vi "eveDataConverter.vi"() -> ()   [LabVIEW 2019]
uses:
  <vilib>/Analysis/NI_AALBase.lvlib
panel:
  out "key sort":u32[](array[numeric])
  out "Value sort":u32[](array[numeric])
  out "Array 2":u32[](array[numeric])
  out "Counts (map)":map{u32, u32}(c390)
  out "Histogram Graph":T1(graph)
  out "Channel":u32[](array[numeric])
  out "Energy":u32[](array[numeric])
  out "Chan+Energy":u32[](array[numeric])
  out "Clk Ticks":u32[](array[numeric])
  out "Sr No":i32[](array[numeric])
  out "Array":string[](array[string])
  out "rsvd+partity":u32
  out "pha":u32
  out "channel":u32
  in  "Input Binary String":string
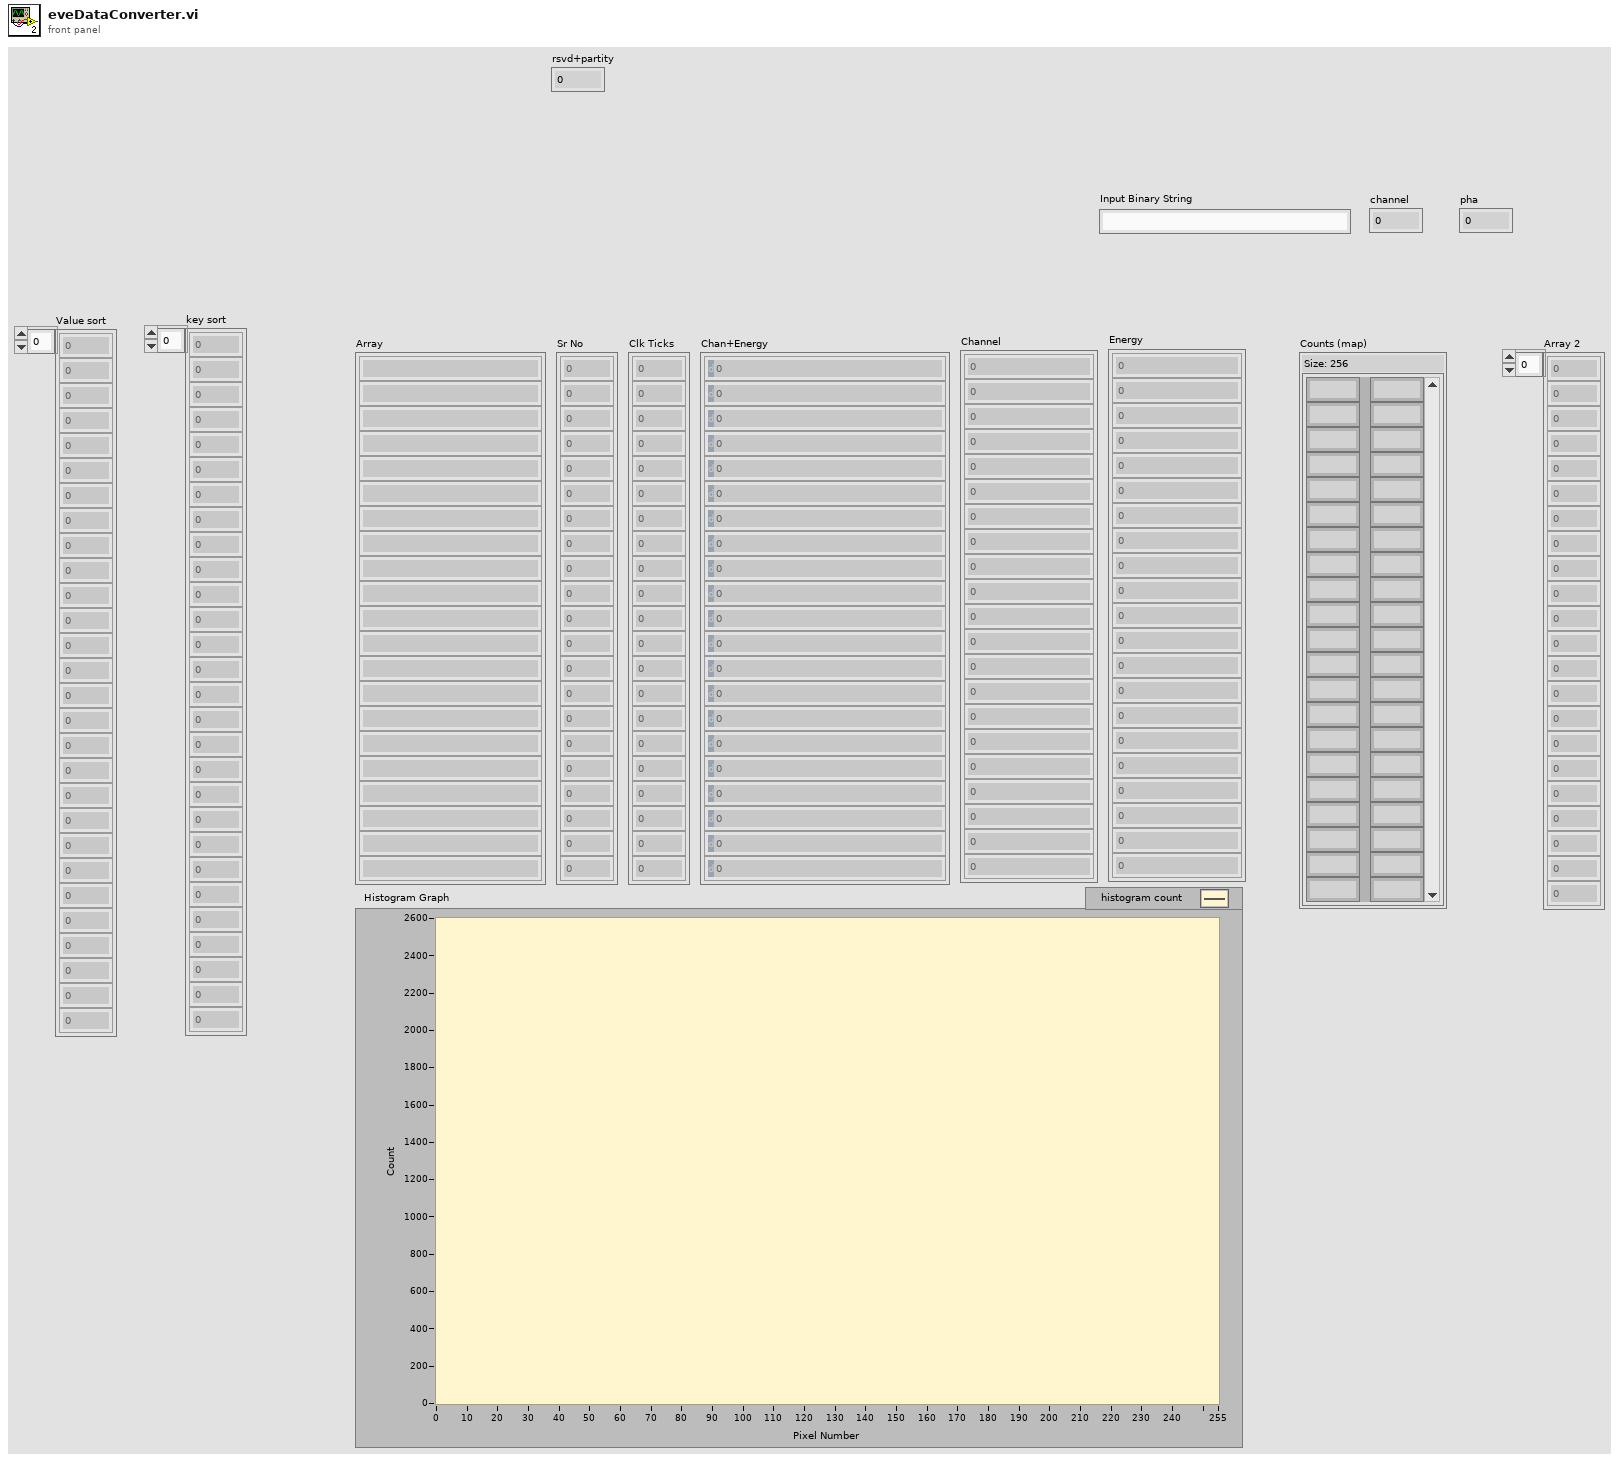
[diagram p1: front panel]
types:
  T1 = cluster{"X Values":dbl[], "Histogram: h(x)":i32[]}
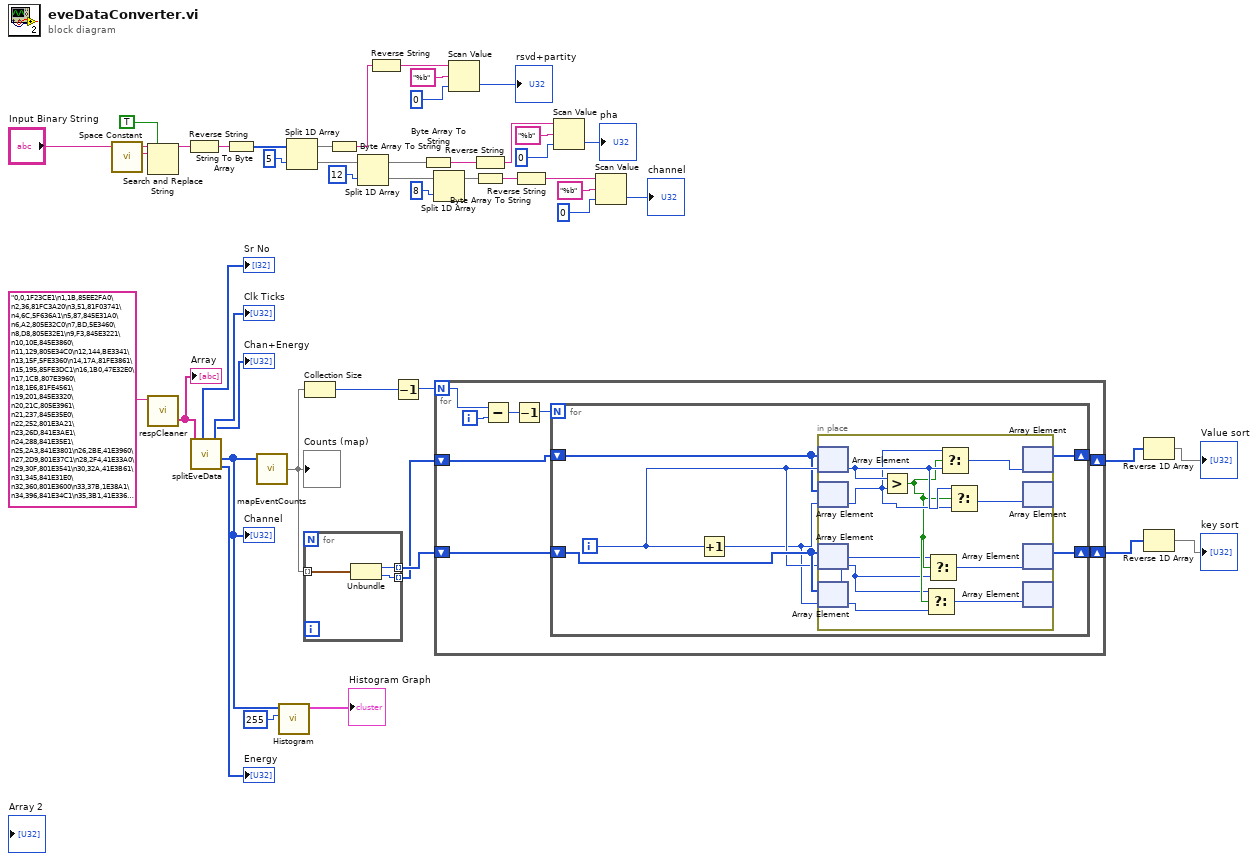
[diagram p0: block diagram]
diagram:
  n1 = call <vilib>:"Space Constant.vi"() -> ("String"=w46:string)
  n2 = Search and Replace String(replace all?=TRUE ("replace all? (F)"), input string="Input Binary String", search string=w46) -> (result string=w41:string)  [unwired: 5 in, 3 out]
  n3 = call "respCleaner.vi"("Raw Response"="0,0,1F23CE1\n1,1B,85EE2FA0\n2,36,81FC3A20\n3,51,81F03741\n4,6C,5F636A1\n5,87,845E31A0\n6,A2,805E32C0\n7,BD,5E3460\n8,D8,805E32E1\n9,F3,845E3221\n10,10E,845E3860\n11,129,805E34C0\n12,144,BE3341\n13,15F,5FE3360\n14,17A,81FE3861\n15,195,85FE3DC1\n16,1B0,47E32E0\n17,1CB,807E3960\n18,1E6,81FE4561\n19,201,845E3320\n20,21C,805E3961\n21,237,845E35E0\n22,252,801E3A21\n23,26D,841E3AE1\n24,288,841E35E1\n25,2A3,841E3801\n26,2BE,41E3960\n27,2D9,801E37C1\n28,2F4,41E33A0\n29,30F,801E3541\n30,32A,41E3B61\n31,345,841E31E0\n32,360,801E3600\n33,37B,1E38A1\n34,396,841E34C1\n35,3B1,41E3360\n36,3CC,801E37C1\n37,3E7,41E3500\n38,402,1E43C1\n39,41D,41E3C41\n40,438,41E36A0\n41,453,801E34C1\n42,46E,41E3541\n43,489,41E3941\n44,4A4,41E37A1\n45,4BF,841E3300\n46,4DA,1E36A0\n47,4F5,801E3880\n48,510,1E3440\n49,52B,1E3FC0\n50,546,1E3641\n51,561,41E3720\n52,57C,801E3720\n53,597,80BE32E0\n54,5B2,80BE35E1\n55,5CD,84BE3161\n56,5E8,84BE34C1\n57,603,4BE3220\n58,61E,80BE30C0\n59,639,1FE3240\n60,654,1FE33C0\n61,66F,7E3681\n62,68A,47E3921\n63,6A5,845E33C1\n64,6C0,45E31C0\n65,6DB,5E3D00\n66,6F6,BE3101\n67,711,4BE36E1\n68,72C,84BE3541\n69,747,5FE3140\n70,762,1FE2F61\n71,77D,85FE33A0\n72,798,81FE3401\n73,7B3,5FE3461\n74,7CE,847E35C0\n75,7E9,7E39A0\n76,804,805E34A0\n77,81F,805E2F81\n78,83A,45E31C0\n79,855,1E40E0\n80,870,801E3641\n81,88B,41E35E1\n82,8A6,841E3B61\n83,8C1,841E3600\n84,8DC,1E3360\n85,8F7,801E3880\n86,912,1E33C0\n87,92D,1E35E1\n88,948,841E35C0\n89,963,1E3960\n90,97E,801E3880\n91,999,1E3660\n92,9B4,801E3560\n93,9CF,801E2FE0\n94,9EA,801E38C1\n95,A05,41E3AC0\n96,A20,1E3560\n97,A3B,801E3AA0\n98,A56,801E3180\n99,A71,1E4380\n100,A8C,1E37A1\n101,AA7,841E40A1\n102,AC2,841E3D61\n103,ADD,84DE38E0\n104,AF8,801E37C1\n105,B13,41E33A0\n106,B2E,801E35E1\n107,B49,841E36C0\n108,B64,1E37C1\n109,B7F,41E3EE0\n110,B9A,801E3A00\n111,BB5,1E34A1\n112,BD0,841E37E0\n113,BEB,801E3C81\n114,C06,41E3CE1\n115,C21,841E3740\n116,C3C,1E3801\n117,C57,41E37E0\n118,C72,801E3521\n119,C8D,841E34C1\n120,CA8,45E2B01\n121,CC3,45E3501\n122,CDE,4BE3360\n123,CF9,80BE32C1\n124,D14,4BE3180\n125,D2F,BE3321\n126,D4A,85FE3740\n127,D65,1FE3201\n128,D80,5FE3261\n129,D9B,85FE30C0\n130,DB6,7E3820\n131,DD1,805E39E0\n132,DEC,80BE3201\n133,E07,4BE3321\n134,E22,84BE35A0\n135,E3D,80BE3261\n136,E58,84BE38A1\n137,E73,85FE3880\n138,E8E,1FE37A1\n139,EA9,85FE33C0\n140,EC4,7E3600\n141,EDF,7E3621\n142,EFA,845E3080\n143,F15,5E3221\n144,F30,841E39A0\n145,F4B,801E3701\n146,F66,41E32E0\n147,F81,801E3120\n148,F9C,801E3740\n149,FB7,1E3761\n150,FD2,841E34E0\n151,FED,801E36E1\n152,1008,841E3BE0\n153,1023,801E38E0\n154,103E,801E37E0\n155,1059,801E3801\n156,1074,41E3641\n157,108F,41E3720\n158,10AA,801E37E0\n159,10C5,801E3621\n160,10E0,841E3500\n161,10FB,1E3CA0\n162,1116,801E3761\n163,1131,841E3761\n164,114C,841E36C0\n165,1167,1E3621\n166,1182,841E3D40\n167,119D,1E3880\n168,11B8,1E35E1\n169,11D3,841E3BC1\n170,11EE,41E3420\n171,1209,801E36E1\n172,1224,841E3280\n173,123F,1E35C0\n174,125A,1E3AA0\n175,1275,80BE3420\n176,1290,80BE3000\n177,12AB,BE3300\n178,12C6,BE3300\n179,12E1,BE3560\n180,12FC,81FE3621\n181,1317,847E3461\n182,1332,845E3421\n183,134D,841E3381\n184,1368,41E37A1\n185,1383,845E3141\n186,139E,41E38E0\n187,13B9,801E35A0\n188,13D4,801E3C60\n189,13EF,801E37C1\n190,140A,41E3560\n191,1425,801E3EE0\n192,1440,801E36E1\n193,145B,841E35E1\n194,1476,841E35C0\n195,1491,1E3480\n196,14AC,1E3521\n197,14C7,841E33A0\n198,14E2,80BE31E0\n199,14FD,80BE32E0\n200,1518,80BE30A0\n201,1533,80BE3280\n202,154E,BE35A0\n203,1569,80BE3440\n204,1584,1FE3261\n205,159F,85FE31E0\n206,15BA,81FE3941\n207,15D5,47E35E1\n208,15F0,845E3481\n209,160B,45E3520\n210,1626,80BE3461\n211,1641,85FE3921\n212,165C,84BE3321\n213,1677,84BE3120\n214,1692,81FE33C0\n215,16AD,1FE3AA0\n216,16C8,81FE3921\n217,16E3,85FE39A0\n218,16FE,807E33E1\n219,1719,841E37E0\n220,1734,805E32A0\n221,174F,805E3160\n222,176A,805E32E1\n223,1785,841E3AE1\n224,17A0,845E3421\n225,17BB,84BE3461\n226,17D6,847E29A1\n227,17F1,84BE3461\n228,180C,84BE3461\n229,1827,85FE33C0\n230,1842,1FE4241\n231,185D,5FE3500\n232,1878,7E3560\n233,1893,805E35E0\n234,18AE,805E34A0\n235,18C9,80BE32A1\n236,18E4,84BE3201\n237,18FF,4BE3360\n238,191A,81FE33E1\n239,1935,85FE35E1\n240,1950,847E3480\n241,196B,5E36C1\n242,1986,45E3320\n243,19A1,805E3601\n244,19BC,4BE3201\n245,19D7,4BE3341\n246,19F2,4BE3480\n247,1A0D,1FE3761\n248,1A28,847E35A0\n249,1A43,81FE4400\n250,1A5E,5E3320\n251,1A79,805E3421\n252,1A94,84BE3541\n253,1AAF,4BE35A0\n254,1ACA,80BE3641\n255,1AE5,5FE3480\n256,1B00,1FE3541\n257,1B1B,5EC3581\n258,1B36,5F047C1\n259,1B51,5EE3800\n260,1B6C,1FA40A0\n261,1B87,81F445C1\n262,1BA2,5F83E20\n263,1BBD,81F64140\n264,1BD8,1FC4180\n265,1BF3,1F24BC0\n266,1C0E,DE39A0\n267,1C29,81FE6EA1\n268,1C44,85FE38A1\n269,1C5F,85FE36C0\n270,1C7A,1FE3600\n271,1C95,1FE30E1\n272,1CB0,85FE3AE1\n273,1CCB,85FE3C21\n274,1CE6,85FE34C1\n275,1D01,5FE37E0\n276,1D1C,81FE4020\n277,1D37,80DE32C1\n278,1D52,5FE4301\n279,1D6D,5FE3D01\n280,1D88,5FE4881\n281,1DA3,47E38E0\n282,2870,1803060\n283,2949,1802EA0\n284,2DE8,1803021\n285,2E93,1803300\n286,39C8,5E32E1\n287,3DEB,1E36E1\n288,3FB2,1E3861\n289,3FE3,1E3A00\n290,402C,DE32C1\n291,405D,1E3B01\n292,40DC,1E41A0\n293,4125,1E3420\n294,4168,1E40E0\n295,41A7,1E3641\n296,41DA,1E38E0\n297,420B,1E3A60\n298,4248,1E3AA0\n299,427D,1E3E01\n300,42B0,DE33E1\n301,42E1,D03460\n302,4314,1E4221\n303,4345,DE3780\n304,4378,1E3560\n305,43CD,1E3801\n306,4400,1E3D61\n307,443F,1E47E1\n308,4472,DE3900\n309,44A9,1E4C01\n310,44E6,1E3CC0\n311,4551,1E3DE0\n312,7E94,BE3101\n313,7FBB,BE3381\n314,835C,1E4B81\n315,8475,1E3740\n316,84F8,1E3921\n317,853F,1E36E1\n318,95CA,5E3301\n319,10427,1FE3581\n320,10472,DE3000\n321,104A3,1FE3A60\n322,104F4,1FE37A1\n323,10543,1FE34C1\n324,10592,1FE3660\n325,1B345,BE3261\n326,1B38E,BE33A0\n327,3218F,1FE3480\n328,321C2,1FE34C1\n329,32211,1FE40A1\n330,32244,1FE3381\n331,3228F,1FE4340\n332,322DE,1FE4620\n333,32329,7E35A0\n334,3235C,1FE4EC0\n335,32395,1FE3861\n336,323C8,DE32A1\n337,323F9,1FE35C0\n338,3242C,7E3720\n339,3245D,1FE34A1\n340,32490,7E3780\n341,324C1,1FE3641\n342,32530,1FE4BA0\n343,34D23,5E3121\n344,34EA4,5E30A1\n345,34F51,5E30E0\n346,34FB0,5E26A0\n347,350A1,5E34A0\n348,35F3A,1E3C00\n349,35FE1,1E35E1\n350,3602A,1E36E1\n351,36073,1E3801\n352,360BC,1E3DC1\n353,36163,1E37A1\n354,361AA,1E3CA0\n355,361F1,1E3440\n356,3623A,1E3E61\n357,36281,1E4100\n358,362BC,1E4080\n359,36305,1E36A0\n360,36338,1E3681\n361,36387,1E35A0\n362,363E4,1E3BE0\n363,36421,1E3681\n364,36470,1E4760\n365,364A5,1E37A1\n366,364EE,1E43C1\n367,36535,1E3C21\n368,36574,1E3981\n369,365DB,1E3780\n370,3662C,1E3C81\n371,36661,1E3461\n372,366B2,1E3F00\n373,366F9,1E3861\n374,3672C,1E3A60\n375,36775,1E3321\n376,367A8,1E3C81\n377,367E1,1E3FA0\n378,368E2,1E34E0\n379,36965,1E37E0\n380,36998,1E4540\n381,36A1D,1E3720\n382,36B62,1E3960\n383,36BFD,1E3BC1\n384,36C68,1E3740\n385,36DD5,1E39A0\n386,36E3A,1E3000\n387,36EAB,1E36A0\n388,36EDE,1E3921\n389,36F0F,DE3880\n390,36F42,1E3F00\n391,36F7B,1E38A1\n392,36FB8,1E3641\n393,36FE9,1E3021\n394,37038,DE3C41\n395,370A7,1E42A0\n396,37104,1E3220\n397,3730D,1E3740\n398,3737C,1E35C0\n399,373FD,1E3C00\n400,37466,1E37A1\n401,37637,1E3B61\n402,3767E,1E35C0\n403,376C7,1E3F21\n404,3778C,1E36A0\n405,377D3,1E35A0\n406,37844,1E3BE0\n407,3794D,1E3440\n408,379BE,1E37A1\n409,37A07,1E43C1\n410,37A3A,1E33C0\n411,37A79,1E3820\n412,37AC2,1E38A1\n413,37B09,1E3F41\n414,37B3C,1E3AA0\n415,37B8B,1E38C1\n416,37BC0,1E3960\n417,37BF1,1E3A21\n418,37C40,DE3521\n419,37C87,1E3A21\n420,37CBA,1E35A0\n421,37D03,1E3A00\n422,37D36,1E34E0\n423,37DDB,1E33E1\n424,38C72,BE33C0\n425,38D5F,BE33C0\n426,48DBE,BE30A0\n427,48E69,BE3600\n428,48EE6,BE3180\n429,4902B,BE34E0\n430,49072,BE33C0\n431,4927B,BE3360\n432,62FC4,1FE3521\n433,63011,7E3A41\n434,63044,1FE36A0\n435,63075,7E3560\n436,630A8,1FE3461\n437,630DF,1FE3DC1\n438,63114,1FE38E0\n439,63149,1FE3CA0\n440,6317C,DE3F41\n441,631AD,1FE3C00\n442,631E4,1FE3D20\n443,63217,1FE5060\n444,6324C,1FE3F21\n445,63299,DE36A0\n446,65BB6,5E33C1\n447,65C47,5E3320\n448,65DBA,5E3680\n449,66105,1E3981\n450,6630C,1E4020\n451,6633D,1E3420\n452,6644A,1E3701\n453,6647B,1E33C0\n454,664F8,1E3581\n455,66529,1E3360\n456,6657A,1E3820\n457,665C3,1E3AE1\n458,66632,1E37A1\n459,66679,1E38C1\n460,666C2,1E3F00\n461,666FD,1E3B61\n462,66730,1E4200\n463,66783,1E3DE0\n464,667B6,1E3780\n465,66805,1E40C1\n466,6685A,1E37C1\n467,668A1,1E3D80\n468,668FA,1E3CC0\n469,66931,1E3A81\n470,6697A,1E3A81\n471,669B1,1E3900\n472,669FC,1E42E1\n473,66A79,1E4421\n474,66AF4,1E3BC1\n475,66B31,1E4121\n476,69040,1E3581\n477,69181,1E3BE0\n478,691FA,1E3D20\n479,6925B,1E3A81\n480,6928E,1E3500\n481,69331,1E3461\n482,69CAA,BE33C0\n483,6A3E7,5E3221\n484,6A5A0,5E3260\n485,71B01,1FE3541\n486,71B4A,1FE3E80\n487,71B91,1FE34C1\n488,71BD8,1FE3701\n489,79D19,BE3180\n490,79DF0,BE3120\n491,93B05,1FE3420\n492,93B46,1FE3440\n493,93B8D,1FE4040\n494,93BD8,1FE3D01\n495,93C23,1FE3440\n496,93C56,1FE38A1\n497,93C95,1FE32E0\n498,93CC8,1FE3981\n499,93CF9,DE3B61\n500,93D2C,1FE3761\n501,93D63,1FE3CE1\n502,93D96,7E3280\n503,93DC7,1FE3BA1\n504,93E1A,DE34E0\n505,93E4B,1FE46C1\n506,96888,5E3281\n507,96B85,5E3481\n508,96BD8,5E3741\n509,971F3,1E3B20\n510,97226,1E3720\n511,97303,1E3B61\n512,9734C,1E33E1\n513,97393,1E3B80\n514,9741E,1E3321\n515,9745D,1E3581\n516,974A6,1E3900\n517,974E5,1E3480\n518,9755A,1E3480\n519,9758B,1E3C81\n520,975BE,DE30A0\n521,97607,1E3600\n522,97650,1E3581\n523,97681,1E3941\n524,976CC,1E40A1\n525,976FD,1E3381\n526,9774E,1E3880\n527,9777F,1E39A0\n528,977C8,1E4B41\n529,977F9,1E36A0\n530,97904,1E3541\n531,97935,1E3840\n532,97972,1E3740\n533,979B3,DE37A1\n534,979F2,1E4640\n535,97B1D,1E4241\n536,97D30,1E4181\n537,99A9F,1E3CA0\n538,99AD8,1E3440\n539,99B21,1E37E0\n540,99B5A,1E32E0\n541,99B8B,1E3581\n542,99BDA,1E3720\n543,99C23,1E3CC0\n544,99CAA,1E36A0\n545,99CF9,1E3541\n546,99D56,1E3B40\n547,9ABE7,BE3161\n548,9AC2A,BE3521\n549,9AC6D,BE3560\n550,9ACA2,BE3360\n551,A2907,1FE3F60\n552,A294A,1FE3681\n553,A297B,1FE3641\n554,A29C4,DE34A1\n555,A29F5,1FE3660\n556,AAD2E,BE33E1\n557,AAD9D,BE3600\n558,AAE54,BE3440\n559,C4991,1FE35A0\n560,C49DC,1FE4141\n561,C4A23,1FE43C1\n562,C4A62,1FE33A0\n563,C4AA9,1FE4481\n564,C4AF0,1FE40C1\n565,C4B21,1FE3060\n566,C4B54,1FE3641\n567,C4B8D,1FE3701\n568,C4BC0,7E3621\n569,C4BF1,1FE35E1\n570,C4C24,DE4260\n571,C4C55,1FE4481\n572,C4C90,1FE46C1\n573,C79E7,5E34E1\n574,C7B26,5E3380\n575,C7C0B,5E3421\n576,C7F12,1E3581\n577,C7F5B,1E3BC1\n578,C7FA4,1E3560\n579,C8163,1E3321\n580,C8196,1E35A0\n581,C81DD,1E3921\n582,C8210,1E39C0\n583,C8259,1E3E20\n584,C82A0,1E3C60\n585,C82E7,1E37E0\n586,C8330,1E4141\n587,C8371,1E35C0\n588,C83BA,1E3820\n589,C83F1,1E3A00\n590,C8492,1E3780\n591,C850D,1E39A0\n592,C8540,1E3B40\n593,C8581,1E39E1\n594,C85B8,1E3BA1\n595,C85FF,DE3DA1\n596,C8640,1E3921\n597,C8671,1E4200\n598,C8758,1E41E1\n599,C87AB,1E4281\n600,C8800,1E4260\n601,C8871,1E4181\n602,C8BCE,1E4901\n603,CA84D,1E3780\n604,CA8B8,1E35C0\n605,CA92F,1E3C00\n606,CA9A0,1E3B20\n607,CA9E7,DE3461\n608,CAA8C,1E47E1\n609,CAACB,1E3A41\n610,CAC60,1E37C1\n611,CB9A1,BE3360\n612,DB98C,BE3220\n613,DB9D7,BE3220\n614,DBAD0,BE3280\n615,F5513,1FE37A1\n616,F5562,1FE3A60\n617,F55B1,1FE3880\n618,F5600,1FE3480\n619,F564B,1FE3820\n620,F5696,1FE4141\n621,F56DD,1FE4EE1\n622,F5728,1FE3EA1\n623,F5773,1FE3EE0\n624,F57BC,1FE3861\n625,F57F5,1FE3461\n626,F5834,1FE35A0\n627,F5865,1FE3220\n628,F5898,DE3801\n629,F58C9,1FE35A0\n630,F58FC,7E33C0\n631,F592D,1FE3701\n632,F596C,1FE4281\n633,F599D,7E3641\n634,F59D0,1FE4260\n635,F5A01,DE3CA0\n636,F5A34,1FE4640\n637,F5A9D,1FE4561\n638,F842C,5E3020\n639,F85E1,5E3B81\n640,F8DAC,1E3861\n641,F931F,1E3701\n642,F9352,1E3BE0\n643,F947B,1E41C0\n644,F94AE,1E3641\n645,F9565,1E3B80\n646,F9598,1E3CA0\n647,F95D1,1E34C1\n648,F9612,1E3621\n649,F9661,1E4020\n650,F9694,1E3CE1\n651,F96EF,1E3560\n652,F974C,1E39E1\n653,F977D,1E3681\n654,F97C6,1E3A41\n655,F98B5,1E3681\n656,F991E,1E3CE1\n657,F999B,1E40A1\n658,F9A08,1E3F81\n659,F9A49,1E3C00\n660,F9A7C,1E41A0\n661,F9AAD,DE3820\n662,F9B22,1E3761\n663,F9B8B,1E3B01\n664,F9BD4,DE3541\n665,FA3B1,1E40C1\n666,FA578,1E3F41\n667,FA8A5,1E3660\n668,FA944,1E4540\n669,FA9AB,1E2C01\n670,FAB9E,1E3960\n671,FABCF,1E33A0\n672,FACB4,1E3621\n673,FAE2B,1E4221\n674,FAEA2,1E3A60\n675,FAF91,1E3420\n676,FB084,1E3820\n677,FB1AD,1E3FA0\n678,FB1E0,1E3660\n679,FB22F,1E3720\n680,FB39C,1E32E0\n681,FB52D,1E35A0\n682,FC632,BE37C1\n683,FC6A9,BE35A0\n684,10CCA2,BE3240\n685,10CDDB,BE3401\n686,10CF1C,BE3261\n687,10D5C7,BE3600\n688,1264F0,1FE3480\n689,126533,1FE3AC0\n690,12657E,1FE4721\n691,1265BF,1FE40E0\n692,1265F2,1FE3641\n693,126623,1FE3DA1\n694,126656,7E37A1\n695,126687,1FE39C0\n696,1266BA,DE3960\n697,1266EB,7E2CA1\n698,12671E,1FE4A20\n699,12676B,DE31C1\n700,129218,5E35A1\n701,129261,5E30E0\n702,1292C0,5E30C1\n703,129307,5E32A0\n704,129344,5E2F60\n705,129375,5E3520\n706,1293C4,5E3EC0\n707,129ACD,1E3740\n708,129C98,1E35C0\n709,129D47,1E3660\n710,129DA4,1E3CE1\n711,129F45,1E37C1\n712,12A020,1E3801\n713,12A05F,1E3681\n714,12A0A2,1E3C41\n715,12A0E9,1E44A0\n716,12A11C,1E3D80\n717,12A157,1E3761\n718,12A1A0,DE34E0\n719,12A1D1,1E38A1\n720,12A246,1E3820\n721,12A277,1E3F41\n722,12A2AA,1E3600\n723,12A2DB,1E3681\n724,12A30E,DE40E0\n725,12A33F,1E3DC1\n726,12A386,1E43A1\n727,12A465,1E3E61\n728,12A4AE,1E40C1\n729,12A4F7,1E40A1\n730,12A52A,1E3440\n731,12A56B,1E39A0\n732,12A5AE,DE3621\n733,12A611,1E41E1\n734,12A7D4,1E4460\n735,12B817,1E4680\n736,12B88C,1E35C0\n737,12BA43,1E41E1\n738,12BD38,1E3A60\n739,12BD7F,DE31E0\n740,12BDDC,1E36E1\n741,12BE0D,1E38A1\n742,12BE54,1E4141\n743,12BE85,1E3480\n744,12BECE,DE3BA1\n745,12BF29,1E3CA0\n746,12C094,1E33A0\n747,12C0DF,1E41E1\n748,12C134,1E3660\n749,12C165,1E3621\n750,12C1D2,1E3840\n751,12C219,1E3A81\n752,12C262,1E3660\n753,12C395,1E3820\n754,12C3C8,1E2A40\n755,12D3D1,BE32E0\n756,12D516,BE36C0\n757,12D585,BE3660\n758,13D95C,BE33E1\n759,13D9A3,BE36C0\n760,13DA4C,BE3A81\n761,13DAB9,BE31A1\n762,13DAFC,BE3941\n763,13DBB9,BE34E0\n764,13DCE8,BE31A1\n765,1571EF,1FE34C1\n766,157236,1FE3BA1\n767,157271,1FE3581\n768,1572BA,1FE4721\n769,1572EB,1FE3C81\n770,157326,1FE32E0\n771,157361,1FE3DA1\n772,1573AC,1FE4721\n773,1573DD,1FE3641\n774,157410,7E36A0\n775,157441,1FE4020\n776,157474,DE3701\n777,1574A5,1FE3761\n778,1574D8,7E3541\n779,157509,1FE41E1\n780,157554,DE36E1\n781,15A0C9,5E32C0\n782,15A11A,5E3340\n783,15A189,5E3281\n784,15A670,1E3C00\n785,15A76B,1E3740\n786,15A81A,1E35A0\n787,15AB7B,1E3A41\n788,15ACFA,1E3A41\n789,15AD3F,1E3E40\n790,15AD8E,1E3B20\n791,15ADEB,1E4320\n792,15AE36,1E48C0\n793,15AE7D,1E4821\n794,15AF08,1E35E1\n795,15AF57,1E3720\n796,15AF9A,1E3581\n797,15AFCB,1E3521\n798,15AFFE,1E3861\n799,15B02F,1E37C1\n800,15B066,1E39E1\n801,15B14B,1E3600\n802,15B1BC,1E39C0\n803,15B331,1E39E1\n804,15B364,1E3F00\n805,15B395,DE3341\n806,15B3C8,1E3761\n807,15B55F,1E5321\n808,15B606,1E4121\n809,15C907,1E3480\n810,15C94A,1E3A41\n811,15CAEB,1E4040\n812,15CC74,1E3F81\n813,15CD19,1E3541\n814,15CDB0,1E3B20\n815,15CDEF,1E41A0\n816,15CE22,1E35E1\n817,15CECB,1E35A0\n818,15CF1A,1E3CE1\n819,15CFB9,1E3A60\n820,15D054,1E3720\n821,15D091,1E3541\n822,15D16E,1E3740\n823,15D1B7,1E3621\n824,15D1FA,1E3480\n825,15E1BF,BE3420\n826,165EEC,1FE3521\n827,165F35,1FE3581\n828,165F86,1FE3960\n829,165FCF,1FE3381\n830,16E2F4,BE3401\n831,16E361,BE3BE0\n832,16E3A2,BE34A1\n833,16E455,BE3360\n834,187F58,1FE3381\n835,187FDD,1FE32E0\n836,188010,1FE32E0\n837,188041,1FE3681\n838,188074,7E3960\n839,1880A5,1FE3900\n840,1880D8,DE33E1\n841,188109,7E3801\n842,18813C,1FE3C41\n843,188177,1FE3C21\n844,1881AA,1FE36C0\n845,1881E3,1FE4AC1\n846,188216,DE4121\n847,18AEF3,5E31E1\n848,18AFE6,5E3441\n849,18B349,1E3440\n850,18B806,1E3AE1\n851,18B855,1E3541\n852,18BA0E,1E39A0\n853,18BAC1,1E3DE0\n854,18BB0A,1E4C01\n855,18BB5B,1E3720\n856,18BBB4,1E3401\n857,18BC01,1E3F81\n858,18BC44,1E37A1\n859,18BC8B,1E3B40\n860,18BCC6,1E3E40\n861,18BD15,1E3761\n862,18BD72,1E3D80\n863,18BDB9,1E37A1\n864,18BE0A,1E3900\n865,18BE3B,1E37A1\n866,18BE72,1E34C1\n867,18BEB3,1E3E40\n868,18BEE6,DE3500\n869,18BF17,1E3880\n870,18BF60,1E3960\n871,18BFA7,1E3F41\n872,18BFF0,1E3D61\n873,18C021,1E3720\n874,18C07A,1E3D01\n875,18C0FB,1E45A1\n876,18C168,1E3960\n877,18C1A7,1E3C41\n878,18C1DA,1E3AC0\n879,18CB95,1E4181\n880,18CDEA,1E45E0\n881,18CE1B,1E3BE0\n882,18D4E6,1E3780\n883,18D65B,1E3CA0\n884,18D6D6,1E4080\n885,18D71F,1E40A1\n886,18D762,1E3AC0\n887,18D793,1E37E0\n888,18D7CE,1E3BA1\n889,18D7FF,DE3740\n890,18D84E,1E3641\n891,18D895,1E4001\n892,18D8E8,1E3A21\n893,18D9D7,1E3600\n894,18DAA2,1E3521\n895,18DAE9,1E3381\n896,18DB3A,1E37A1\n897,18DBF3,1E3401\n898,18DCF6,1E3D40\n899,18DD3F,1E3621\n900,18DF58,1E38E0\n901,18EE57,BE3621\n902,18EEFC,BE3240\n903,18F3B5,5E3361\n904,1957C8,7E3480\n905,196C2B,1FE3440\n906,196CA2,1FE32E0\n907,196CF1,1FE3BE0\n908,196D40,1FE3B40\n909,19F45B,BE26A1\n910,19F4F6,BE3321\n911,19F563,BE3461\n912,19F5A6,BE31E0\n913,19F60F,BE3720\n914,19F78E,BE36E1\n915,19F8C5,BE36A0\n916,1B8D46,1FE37C1\n917,1B8DCB,1FE3401\n918,1B8E16,1FE4441\n919,1B8E47,1FE3C21\n920,1B8E90,1FE43A1\n921,1B8EC1,7E3401\n922,1B8EF4,1FE3C60\n923,1B8F2F,1FE3CC0\n924,1B8F62,1FE3B61\n925,1B8F93,DE3420\n926,1B8FC6,7E35E1\n927,1B8FF7,7E35C0\n928,1B902A,1FE4181\n929,1BBCC5,5E36E0\n930,1BC752,1E3600\n931,1BC845,1E43C1\n932,1BC88E,DE3440\n933,1BC8BF,1E4AA1\n934,1BC8FC,1E33C0\n935,1BC945,1E34E0\n936,1BCA0C,1E38C1\n937,1BCA3D,1E35A0\n938,1BCA9A,1E3681\n939,1BCACB,1E3780\n940,1BCB52,1E3740\n941,1BCBA9,1E36E1\n942,1BCBEC,1E3740\n943,1BCC35,1E38A1\n944,1BCC68,1E4260\n945,1BCCA3,1E3D20\n946,1BCCE6,1E3F00\n947,1BCD2D,1E3941\n948,1BCD76,1E3E20\n949,1BCDB1,1E37A1\n950,1BCDE4,1E35E1\n951,1BCE15,1E3861\n952,1BCE8E,1E38C1\n953,1BCECD,1E3C21\n954,1BCF0E,DE3E80\n955,1BCF3F,1E4800\n956,1BCF78,1E3820\n957,1BCFC7,1E3FA0\n958,1BD008,1E3FA0\n959,1BD075,1E3A60\n960,1BD15A,1E4061\n961,1BD1D1,1E3480\n962,1BD4DA,1E3D40\n963,1BE20F,1E34C1\n964,1BE2B6,1E46C1\n965,1BE2FD,1E3BE0\n966,1BE34C,1E3F00\n967,1BE4C5,1E29E0\n968,1BE578,1E34E0\n969,1BE5D5,1E2301\n970,1BE646,1E3780\n971,1BE8EF,1E3401\n972,1BE9AE,1E3B61\n973,1BEA2D,1E3C41\n974,1BFC1C,BE3921\n975,1BFC67,BE31E0\n976,1BFCD4,BE3420\n977,1BFD09,BE31E0\n978,1BFD52,DE34C1\n979,1BFF8F,5E31E1\n980,1C794C,1FE3C21\n981,1C7991,1FE3541\n982,1C79D8,1FE4281\n983,1CFE85,BE3A00\n984,1CFF72,BE23E0\n985,1CFFEB,BE3440\n986,1D002E,BE3EE0\n987,1E9817,1FE34C1\n988,1E999C,1FE35A0\n989,1E99E3,1FE3420\n990,1E9A32,1FE3B61\n991,1E9A7B,1FE48C0\n992,1E9AC4,1FE3BE0\n993,1E9AF5,1FE3521\n994,1E9B3C,1FE4281\n995,1E9B71,1FE34E0\n996,1E9BBA,1FE4901\n997,1E9BEB,1FE39E1\n998,1E9C26,7E3360\n999,1E9C57,1FE3E40\n1000,1E9C8A,DE39C0\n1001,1E9CBB,1FE3801\n1002,1E9CF6,1FE4CA1\n1003,1E9D27,1FE4241\n1004,1E9D76,DE35E1\n1005,1EC8EB,5E32C0\n1006,1ECA26,5E31A0\n1007,1ED2DB,1E3780\n1008,1ED318,1E3820\n1009,1ED521,1E36A0\n1010,1ED56E,1E3461\n1011,1ED5BD,1E3701\n1012,1ED658,1E3801\n1013,1ED6A9,1E37C1\n1014,1ED6EC,1E3500\n1015,1ED733,1E3941\n1016,1ED77A,1E3820\n1017,1ED7C1,1E3D40\n1018,1ED808,1E3600\n1019,1ED839,1E3C00\n1020,1ED884,1E4221\n1021,1ED8B5,1E3FC0\n1022,1ED8FC,DE3BE0\n1023,1ED92D,1E3D61\n1024,1ED97E,1E44E1\n1025,1ED9AF,1E34E0\n1026,1ED9EC,1E40A1\n1027,1EDA57,1E44A0\n1028,1EDB88,1E3A81\n1029,1EDBCF,1E4940\n1030,1EDCE4,1E3D20\n1031,1EDD4B,1E4501\n1032,1EDDA4,1E3C00\n1033,1EDE23,1E3F81\n1034,1EF576,1E3A81\n1035,1EF60B,1E3621\n1036,1EF662,1E3621\n1037,1EF6A9,1E3401\n1038,1EF6F0,1E3E20\n1039,1EF739,1E40E0\n1040,1EF78C,1E38E0\n1041,1EF7D5,1E3880\n1042,1EF818,1E36A0\n1043,1EF8CD,1E3DC1\n1044,1EF942,1E3560\n1045,1EFA6B,1E3FC0\n1046,1F09D0,BE31E0\n1047,1F0A49,BE3280\n1048,1F0C10,5E3320\n1049,200F13,BE3801\n1050,2011A6,BE3280\n1051,201215,BE3060\n1052,201322,BE3060\n1053,21A811,1FE3CE1\n1054,21A85C,1FE3720\n1055,21A8A5,1FE40A1\n1056,21A8DA,1FE3101\n1057,21A919,1FE37A1\n1058,21A94C,1FE3960\n1059,21A989,1FE3880\n1060,21A9BC,7E34C1\n1061,21A9ED,1FE3880\n1062,21AA20,DE38A1\n1063,21AA51,7E3C00\n1064,21AA84,1FE4DA0\n1065,21AAB9,1FE4700\n1066,21D696,5E3781\n1067,21D6CB,5E3380\n1068,21D714,DE3981\n1069,21DE53,1E3500\n1070,21DE9C,1E3560\n1071,21DED7,1E3600\n1072,21E018,1E37E0\n1073,21E067,1E3941\n1074,21E0AC,1E3C21\n1075,21E1D3,1E3820\n1076,21E21E,1E3AA0\n1077,21E261,1E4020\n1078,21E35A,1E4DC0\n1079,21E3A1,1E3440\n1080,21E3E8,1E4181\n1081,21E425,1E4421\n1082,21E48E,1E36A0\n1083,21E4D5,1E3740\n1084,21E514,1E39A0\n1085,21E563,1E5220\n1086,21E650,1E44C0\n1087,21E835,1E48E1\n1088,21FF30,1E3A21\n1089,2202AB,1E34C1\n1090,220316,1E3960\n1091,2203EB,1E3D80\n1092,2204DA,1E3461\n1093,220547,1E3641\n1094,220644,1E37C1\n1095,2206E5,1E3660\n1096,22072E,1E3681\n1097,220783,1E36C0\n1098,2207CC,1E35C0\n1099,2217DB,BE33E1\n1100,22184C,BE3521\n1101,229391,1FE38E0\n1102,231A50,BE3220\n1103,231A97,BE32C1\n1104,231AD6,BE3420\n1105,231B81,BE35C0\n1106,231CDE,BE3060\n1107,231E1F,BE3261\n1108,24B666,1FE31C1\n1109,24B697,7E3360\n1110,24B6DE,1FE4F40\n1111,24B70F,7E34A1\n1112,24B742,1FE34A1\n1113,24B777,1FE3A21\n1114,24B7B6,1FE3A41\n1115,24B7E7,DE4760\n1116,24B81A,1FE3BE0\n1117,24B853,1FE4221\n1118,24B8BC,1FE39A0\n1119,24E661,5E3821\n1120,24E6F0,5E3520\n1121,24EA0F,1E3541\n1122,24EBCC,1E3C81\n1123,24ED9D,1E3E80\n1124,24EDE0,1E3F81\n1125,24EE21,DE32C1\n1126,24EE54,1E3341\n1127,24EE85,1E3480\n1128,24EEC8,1E3660\n1129,24EF31,1E3C60\n1130,24EF7A,1E3840\n1131,24EFC3,1E3D61\n1132,24F00C,1E3541\n1133,24F03D,1E4181\n1134,24F0E0,1E3780\n1135,24F117,1E35A0\n1136,24F15E,1E3720\n1137,24F18F,1E3B61\n1138,24F1CC,1E3BA1\n1139,24F1FD,DE3E61\n1140,24F230,1E3E40\n1141,24F297,1E4001\n1142,24F306,1E3DC1\n1143,24F3D7,1E3C41\n1144,24F4C2,1E43C1\n1145,2512C7,1E3600\n1146,25133A,1E4380\n1147,25157D,1E3A41\n1148,2516C4,1E3941\n1149,251743,1E3AE1\n1150,2517E0,1E3840\n1151,252461,BE3401\n1152,25250C,5E32C0\n1153,25254F,BE3861\n1154,2525BA,5E3320\n1155,25A035,1FE3EE0\n1156,25A0C4,1FE36C0\n1157,25A10D,1FE4800\n1158,25A154,1FE3AE1\n1159,25A19B,1FE37C1\n1160,25A1E4,1FE36A0\n1161,262B0B,BE3401\n1162,262B54,BE3C81\n1163,262C03,BE32C1\n1164,262C72,BE3201\n1165,262D5F,BE3201\n1166,262EB8,BE3321\n1167,27C2AF,1FE3321\n1168,27C2F8,1FE4E81\n1169,27C335,1FE3461\n1170,27C37E,1FE43A1\n1171,27C3AF,1FE3DA1\n1172,27C3EC,1FE3981\n1173,27C421,1FE3420\n1174,27C454,DE3F21\n1175,27C485,1FE40C1\n1176,27C4B8,7E3621\n1177,27C4E9,1FE3880\n1178,27C51C,DE34C1\n1179,27C553,1FE39E1\n1180,27C586,1FE4961\n1181,27C5B7,DE3F60\n1182,27EE48,5E3281\n1183,27F01D,5E33A1\n1184,27F894,1E35C0\n1185,27FA0F,1E32E0\n1186,27FA50,1E36A0\n1187,27FC0D,1E3D01\n1188,27FC40,1E3681\n1189,27FCBB,1E37E0\n1190,27FCEE,1E3681\n1191,27FD1F,1E36C0\n1192,27FD52,DE42A0\n1193,27FD83,1E47E1\n1194,27FDBC,1E33E1\n1195,27FE03,1E37A1\n1196,27FE4A,1E3581\n1197,27FE87,1E3C60\n1198,27FED0,1E4061\n1199,27FF01,1E39C0\n1200,27FF98,1E3960\n1201,27FFE1,1E39C0\n1202,28004A,1E3DC1\n1203,28007B,1E4281\n1204,2800BC,1E36E1\n1205,280163,1E3C60\n1206,2801AC,1E4380\n1207,28029D,1E3C00\n1208,28048E,1E3341\n1209,281DAB,1E3461\n1210,281FE8,1E37A1\n1211,282031,1E3381\n1212,282064,1E3720\n1213,282095,1E38A1\n1214,2820C8,1E40E0\n1215,2820F9,DE4001\n1216,28212C,1E44C0\n1217,28323B,BE3060\n1218,283284,BE31C1\n1219,2832FB,BE3060\n1220,292FE4,BE3840\n1221,293095,BE39A0\n1222,2931F0,BE34A1\n1223,29332F,BE3560\n1224,29348E,BE3140\n1225,2935E1,BE3180\n1226,29373C,BE3180\n1227,2ACF3F,1FE3780\n1228,2ACF72,1FE2A01\n1229,2ACFA3,1FE3C21\n1230,2ACFEC,1FE4C20\n1231,2AD01D,1FE3641\n1232,2AD068,1FE3A81\n1233,2AD099,1FE3960\n1234,2AD0CC,DE3761\n1235,2AD0FD,1FE36E1\n1236,2AD148,1FE48C0\n1237,2AD179,1FE3600\n1238,2AD1BA,1FE4141\n1239,2AD1EB,1FE3720\n1240,2AD21E,7E34A1\n1241,2AD24F,1FE3D80\n1242,2AD282,DE43E0\n1243,2AD2B3,7E3461\n1244,2AFE44,5E34C0\n1245,2B0747,1E3681\n1246,2B07F4,1E3660\n1247,2B083B,DE30C0\n1248,2B086E,1E3AE1\n1249,2B08CB,1E38A1\n1250,2B0978,1E3341\n1251,2B09FB,1E3D01\n1252,2B0AC8,1E3720\n1253,2B0B0F,1E3921\n1254,2B0B4C,1E3900\n1255,2B0B7D,1E37C1\n1256,2B0BB0,1E4640\n1257,2B0C0B,1E39E1\n1258,2B0C46,1E3861\n1259,2B0C8B,1E35A0\n1260,2B0CBE,1E3621\n1261,2B0D15,1E3480\n1262,2B0D48,1E3761\n1263,2B0D83,1E41A0\n1264,2B0DB6,DE34A1\n1265,2B0E39,1E3541\n1266,2B0E74,1E39A0\n1267,2B0EBD,DE33E1\n1268,2B0F18,1E3921\n1269,2B105B,1E4040\n1270,2B10B8,1E3D01\n1271,2B284B,1E4561\n1272,2B2A38,1E3981\n1273,2B2B65,1E3641\n1274,2B2BC2,1E3D40\n1275,2B2D53,1E3500\n1276,2B2E68,1E34A1\n1277,2B2EAF,1E3941\n1278,2B2EE4,1E3C00\n1279,2B2F31,1E3A21\n1280,2B2F90,1E3B40\n1281,2B2FD9,1E34E0\n1282,2B300E,1E2A20\n1283,2B305D,1E3C81\n1284,2B30CA,1E36E1\n1285,2B3E5F,BE3440\n1286,2BBC44,1FE3341\n1287,2BBC8B,1FE3621\n1288,2BBCDA,1FE4061\n1289,2C49F5,BE3600\n1290,2C4B46,BE3261\n1291,2DDDB1,1FE32C1\n1292,2DDDFA,1FE4640\n1293,2DDE37,1FE3720\n1294,2DDE7E,1FE4561\n1295,2DDEAF,1FE3541\n1296,2DDEEC,1FE38C1\n1297,2DDF1F,1FE3280\n1298,2DDF52,7E3761\n1299,2DDF83,1FE3621\n1300,2DDFB6,DE33C0\n1301,2DDFE7,1FE3D20\n1302,2DE01A,7E3B61\n1303,2DE04B,1FE4580\n1304,2DE086,1FE4080\n1305,2DE0D1,DE3381\n1306,2E0C0C,5E3340\n1307,2E0C57,5E31E1\n1308,2E0CC6,5E33C1\n1309,2E11EB,1E31C1\n1310,2E1302,1E3641\n1311,2E1333,1E3780\n1312,2E1366,DE3440\n1313,2E13B5,1E3A00\n1314,2E1468,1E37C1\n1315,2E1499,1E3261\n1316,2E14CC,1E3861\n1317,2E150F,1E3420\n1318,2E1556,1E3880\n1319,2E159D,1E45C1\n1320,2E15D0,1E4400\n1321,2E1625,1E4281\n1322,2E1658,1E39A0\n1323,2E16B5,1E3461\n1324,2E16F6,1E3DA1\n1325,2E173D,1E48E1\n1326,2E1786,1E3B61\n1327,2E17CF,1E35A0\n1328,2E1810,1E3EA1\n1329,2E1857,DE33A0\n1330,2E18F8,1E37A1\n1331,2E1929,1E39A0\n1332,2E1962,1E37E0\n1333,2E1993,1E3E61\n1334,2E19C6,DE3FA0\n1335,2E19F7,1E3F81\n1336,2E1A34,1E38C1\n1337,2E1A77,1E3921\n1338,2E1AAA,1E4380\n1339,2E1AF3,DE3621\n1340,2E1BF2,1E39C0\n1341,2E1D2D,1E3981\n1342,2E1D9E,1E4441\n1343,2E1EB1,1E42E1\n1344,2E32A2,1E49E0\n1345,2E3A61,1E2F01\n1346,2E3C32,1E3681\n1347,2E3CA3,1E37E0\n1348,2E3CD6,1E34A1\n1349,2E3D1D,1E3581\n1350,2E3D66,1E3960\n1351,2E3E5B,1E3780\n1352,2E3ECE,1E3A00\n1353,2E3F21,1E3000\n1354,2E4D5A,BE3541\n1355,2F438F,BE33C0\n1356,2F4442,BE3401\n1357,2F4481,BE3F21\n1358,2F468A,BE3801\n1359,2F4805,BE3461\n1360,2F484C,1FE3401\n1361,2F487D,BE3420\n1362,30EA78,1FE31C1\n1363,30EAC1,1FE3DC1\n1364,30EAFC,1FE3A21\n1365,30EB3F,1FE37E0\n1366,30EB72,1FE3500\n1367,30EBB3,7E3300\n1368,30EBE6,1FE47A0\n1369,30EC17,DE4001\n1370,30EC4A,1FE3461\n1371,30EC7B,7E3D20\n1372,30ECAE,1FE3C60\n1373,30ECDF,7E3CA0\n1374,30ED18,1FE3B20\n1375,30ED5D,DE36A0\n1376,30EDC8,1FE3FE1\n1377,311B25,5E32E1\n1378,311D94,1E3880\n1379,31200F,1E36C0\n1380,312098,1E3541\n1381,3122DD,1E3220\n1382,312326,1E37E0\n1383,312371,1E3440\n1384,3123BA,1E32E0\n1385,31241B,1E39E1\n1386,312454,1E3AA0\n1387,312559,1E3740\n1388,312594,1E3801\n1389,3125E3,1E3701\n1390,31261C,1E3AE1\n1391,31264D,1E3BE0\n1392,312680,DE3AC0\n1393,3126B1,1E3C21\n1394,3126E4,1E3A60\n1395,31271D,1E3861\n1396,312760,1E4460\n1397,312791,1E3C41\n1398,3127C4,DE36A0\n1399,312805,1E36E1\n1400,31284E,1E3921\n1401,312895,1E4501\n1402,3128C8,1E3880\n1403,3128FF,1E3801\n1404,312946,1E3DC1\n1405,3129A3,1E3960\n1406,312A12,1E36E1\n1407,312B63,1E37C1\n1408,312C84,1E3DC1\n1409,312EDD,1E4481\n1410,314022,1E4361\n1411,3143A1,1E4061\n1412,3143D4,1E3C21\n1413,314423,1E36A0\n1414,31446C,1E42E1\n1415,3144B3,1E3AE1\n1416,31451E,1E2A40\n1417,31454F,1E3820\n1418,3145F4,1E3521\n1419,314671,1E33C0\n1420,3146F8,1E3981\n1421,31473F,1E45C1\n1422,31477A,1E3461\n1423,3147AF,1E3801\n1424,3147F8,1E3CE1\n1425,314847,1E4160\n1426,3148C2,1E37A1\n1427,314973,1E3401\n1428,315B36,BE3261\n1429,315BA7,BE32A1\n1430,326224,BE2DC0\n1431,32630D,BE3000\n1432,326350,BE3261\n1433,326427,BE33C0\n1434,33F772,1FE31A1\n1435,33F85D,1FE34A1\n1436,33F8A6,1FE3941\n1437,33F8ED,1FE3F21\n1438,33F936,7E3560\n1439,33F967,1FE5021\n1440,33F9A0,1FE3280\n1441,33F9D9,1FE3F60\n1442,33FA0C,DE34E0\n1443,33FA3D,1FE3801\n1444,33FA70,7E3B20\n1445,33FAA1,1FE3641\n1446,33FAD4,7E3681\n1447,33FB05,1FE3CA0\n1448,33FB40,1FE5341\n1449,33FB71,DE3581\n1450,34274A,5E30A1\n1451,34278B,5E3421\n1452,3427D6,5E32A0\n1453,342A6B,1E3581\n1454,342AB4,1802D21\n1455,342FFF,1E3861\n1456,343048,1E3621\n1457,34308B,1E3B01\n1458,34313C,1E3740\n1459,343179,1E3B20\n1460,3431AC,DE3AE1\n1461,3431DD,1E3621\n1462,343210,1E3360\n1463,343251,1E36C0\n1464,343292,1E39C0\n1465,3432CD,1E3500\n1466,343300,DE37E0\n1467,343331,1E3921\n1468,34337A,1E3921\n1469,3433AB,1E3500\n1470,3433F4,1E3A00\n1471,343493,1E45C1\n1472,3434C6,1E3761\n1473,3434FB,1E3960\n1474,343550,1E3BE0\n1475,3435AD,1E3840\n1476,343618,1E3921\n1477,34364D,1E3420\n1478,343684,1E3660\n1479,3436BF,1E3921\n1480,3436F2,DE43A1\n1481,343723,1E3CC0\n1482,34379C,1E3C60\n1483,343843,1E42C0\n1484,3438B4,1E4601\n1485,343D6F,1E50A0\n1486,3454FC,1E3641\n1487,345569,1E4061\n1488,345742,1E3D01\n1489,34577F,1E3E40\n1490,3457C8,1E3621\n1491,345843,1E3600\n1492,345894,1E3C41\n1493,3458DB,1E46C1\n1494,34590E,1E3720\n1495,345955,1E35E1\n1496,3459A4,1E3C41\n1497,3459DF,1E4020\n1498,3467DE,BE3560\n1499,346817,BE3740\n1500,34E3AE,1FE2680\n1501,34E3F7,1FE3E61\n1502,34E43E,1FE4400\n1503,34E485,1FE3960\n1504,356F5C,BE37C1\n1505,3570C9,BE3000\n1506,35720E,BE33A0\n1507,370469,1FE3720\n1508,37061C,1FE35E1\n1509,370667,1FE3D80\n1510,3706B0,1FE49C1\n1511,3706E1,1FE3621\n1512,370722,1FE36E1\n1513,370757,7E33C0\n1514,37078A,1FE3A00\n1515,3707BB,DE3880\n1516,3707EE,1FE3861\n1517,37082B,1FE3521\n1518,370896,1FE4D00\n1519,3734D1,5E32E1\n1520,373594,5E3481\n1521,37362D,5E3340\n1522,373D08,1E34A1\n1523,373DC9,1E3941\n1524,373E12,DE3341\n1525,373E43,1E35E1\n1526,373E76,1E37A1\n1527,373EBD,1E3801\n1528,373F08,1E3C00\n1529,373F65,1E3621\n1530,373F98,1E3461\n1531,373FD9,1E3740\n1532,374088,1E3300\n1533,3740C5,1E3A21\n1534,374104,1E3780\n1535,374135,1E3820\n1536,374168,1E3880\n1537,374199,1E3900\n1538,3741CC,DE31C1\n1539,3741FD,1E45E0\n1540,37424C,1E3621\n1541,374293,1E34A1\n1542,37435C,1E3F41\n1543,3743A3,1E4540\n1544,3743D6,1E3D80\n1545,374429,1E3641\n1546,374472,1E40A1\n1547,3744A3,1E3C00\n1548,3744D6,1E3101\n1549,374515,1E4501\n1550,374548,1E3F00\n1551,374583,1E43A1\n1552,3745CC,DE3AA0\n1553,374695,1E4661\n1554,3761B4,1E3CA0\n1555,37629D,1E3DE0\n1556,376336,1E3681\n1557,3763A7,1E3701\n1558,376464,1E34A1\n1559,3764CB,1E3600\n1560,37654C,1E3A00\n1561,3765BD,1E3280\n1562,3766BE,1E3780\n1563,3767FB,1E3440\n1564,37758E,BE34A1\n1565,377871,5E3800\n1566,37F1C0,1FE3E61\n1567,37F20F,1FE3D80\n1568,37F25A,1FE3420\n1569,37F2A3,1FE3541\n1570,387CC6,BE31A1\n1571,387EB5,BE3900\n1572,387EF2,BE36A0\n1573,387FE1,BE3201\n1574,388288,BE33A0\n1575,3883D9,BE3240\n1576,3A11BA,1FE3521\n1577,3A1203,1FE3FA0\n1578,3A1252,1FE3DA1\n1579,3A1299,1FE3D61\n1580,3A12E4,1FE3F81\n1581,3A132D,1FE49C1\n1582,3A1360,1FE3720\n1583,3A139D,1FE3D20\n1584,3A13D0,1FE3581\n1585,3A140D,1FE4160\n1586,3A1440,DE3D20\n1587,3A1471,1FE3C21\n1588,3A14AA,1FE3DE0\n1589,3A14DB,1FE3BC1\n1590,3A150E,7E35E1\n1591,3A153F,1FE4040\n1592,3A1572,DE33E1\n1593,3A425D,5E32E1\n1594,3A4314,5E3760\n1595,3A435B,5E35A1\n1596,3A4476,1E4121\n1597,3A44A7,18039E1\n1598,3A44DA,5E39A1\n1599,3A4831,1802D60\n1600,3A4880,1E3DA1\n1601,3A48C9,18033A0\n1602,3A493A,1802481\n1603,3A49BD,1E39A0\n1604,3A4AB2,1803000\n1605,3A4AFD,1E3C00\n1606,3A4B30,1802E00\n1607,3A4BC1,1E35C0\n1608,3A4D48,1E36E1\n1609,3A4D91,1802C01\n1610,3A4DC4,1E33E1\n1611,3A4E13,1E3AC0\n1612,3A4E5C,1802E21\n1613,3A4EA3,1E4580\n1614,3A5000,1E3A00\n1615,3A50A9,1E41E1\n1616,3A50F2,1E3AA0\n1617,3A5139,1E4640\n1618,3A516C,18034C1\n1619,3A519D,1E3F60\n1620,3A51D4,1E32C1\n1621,3A5209,1E39E1\n1622,3A5252,DE4080\n1623,3A5283,1E41E1\n1624,3A52BC,1E3861\n1625,3A52FF,1E3740\n1626,3A5348,1E3960\n1627,3A538B,1E35E1\n1628,3A53CC,1E3D61\n1629,3A5413,1E4A61\n1630,3A5446,1E3900\n1631,3A54B7,1E3740\n1632,3A54EA,1E3F60\n1633,3A551B,DE3960\n1634,3A554E,1E3861\n1635,3A55F1,1E35E1\n1636,3A56C6,1E4620\n1637,3A57DB,1E34C1\n1638,3A5852,1E3420\n1639,3A5C3F,1E3EE0\n1640,3A5E16,1E3CE1\n1641,3A60A9,1E39E1\n1642,3A6224,1E42A0\n1643,3A634F,1E3461\n1644,3A64B6,1E38A1\n1645,3A6523,1E42A0\n1646,3A65CC,1E3DC1\n1647,3A65FD,1E35A0\n1648,3A6630,DE3461\n1649,3A668D,1E3720\n1650,3A66C0,1E3E01\n1651,3A6709,1E40A1\n1652,3A673C,1E39E1\n1653,3A6783,DE3560\n1654,3A6848,1E3720\n1655,3A68BB,1E37A1\n1656,3A6922,1E3A00\n1657,3A69CB,1E3641\n1658,3A6AB2,1E3761\n1659,3A6AE3,1E3CC0\n1660,3A6B34,1E3780\n1661,3A6B85,1E3C60\n1662,3A6BCE,1E4061\n1663,3A6C03,1E3B40\n1664,3A6C4C,1E35E1\n1665,3A6E2D,1E3381\n1666,3A6E8A,1E3720\n1667,3A8469,BE3280\n1668,3A84E2,BE36E1\n1669,3B82F7,BE3220\n1670,3B8464,BE3280\n1671,3B85B9,BE31A1\n1672,3B8606,BE3261\n1673,3B86F5,BE3060\n1674,3D1FCA,1FE3280\n1675,3D2011,1FE3761\n1676,3D205A,1FE3E01\n1677,3D20A1,1FE3BA1\n1678,3D20D4,1FE3280\n1679,3D211B,1FE4A01\n1680,3D214E,1FE3581\n1681,3D2187,1FE3AC0\n1682,3D21C4,1FE36A0\n1683,3D21F5,7E34A1\n1684,3D2228,1FE4821\n1685,3D2259,DE43C1\n1686,3D228C,1FE3621\n1687,3D22BD,7E3921\n1688,3D22F0,1FE3840\n1689,3D2321,DE34A1\n1690,3D4E2C,5E3340\n1691,3D4E73,5E3221\n1692,3D4F46,5E3940\n1693,3D4F8F,5E3241\n1694,3D5012,5E30E0\n1695,3D5105,1E3681\n1696,3D5154,1E3DA1\n1697,3D5489,1E3360\n1698,3D54D4,1E33A0\n1699,3D578B,1E3E80\n1700,3D57D2,1E3560\n1701,3D590D,1E3440\n1702,3D5956,1E3440\n1703,3D5A1D,1E3500\n1704,3D5A60,1E3581\n1705,3D5AA7,1E3981\n1706,3D5AF8,1E3EC1\n1707,3D5B37,1E3500\n1708,3D5B80,1E4800\n1709,3D5BC7,1E3AA0\n1710,3D5C02,1E3B20\n1711,3D5C33,1E3AE1\n1712,3D5C66,DE3981\n1713,3D5C97,1E3720\n1714,3D5CDA,1E38A1\n1715,3D5D1D,1E4320\n1716,3D5D60,1E4A80\n1717,3D5DC5,1E3560\n1718,3D5DF8,1E3E20\n1719,3D5E31,1E3B61\n1720,3D5E6E,1E3AC0\n1721,3D5EB7,DE3C21\n1722,3D5EEA,1E3360\n1723,3D5F25,1E4B21\n1724,3D7FBA,1E42A0\n1725,3D8043,1E3740\n1726,3D80A0,1E3AC0\n1727,3D80E1,1E3B40\n1728,3D812C,1E3B40\n1729,3D81CD,1E3521\n1730,3D8270,1E35E1\n1731,3D82A1,1E39A0\n1732,3D82E8,1E3420\n1733,3D8461,1E38A1\n1734,3D90FE,BE32E0\n1735,3E0C8D,1FE3660\n1736,3E9476,BE3440\n1737,3E960F,BE3300\n1738,3E979A,BE33A0\n1739,3E98A9,BE33A0\n1740,3E9A2E,BE32E0\n1741,402DB1,1FE4040\n1742,402DFC,1FE44A0\n1743,402E39,1FE3681\n1744,402E6C,1FE3701\n1745,402EA7,1FE36E1\n1746,402EDC,1FE3341\n1747,402F15,1FE3761\n1748,402F48,1FE3440\n1749,402F79,7E3480\n1750,402FAC,1FE3CA0\n1751,402FDD,DE45E0\n1752,403010,1FE3780\n1753,403041,7E3740\n1754,40308A,7E3521\n1755,4030BB,1FE3E01\n1756,4055B8,1802DE1\n1757,405601,1802D60\n1758,405B9E,1802AC1\n1759,405CA7,5E3601\n1760,405CF0,1802C40\n1761,405F19,1E3CE1\n1762,405F4C,1802FE0\n1763,406287,1E3600\n1764,40632A,1E36E1\n1765,40641F,1E3681\n1766,406468,DE33E1\n1767,406499,1E4421\n1768,4064F6,1E36E1\n1769,406551,1E3BA1\n1770,406584,1E3B61\n1771,4065CB,1802F61\n1772,4065FE,1E3CA0\n1773,406645,1E3A41\n1774,40668E,1E3C00\n1775,4066BF,1E3280\n1776,4066F2,18032E0\n1777,406723,1E3581\n1778,406766,1E3440\n1779,406797,1802D60\n1780,4067D2,1E3AA0\n1781,406811,1E3CE1\n1782,406854,DE3861\n1783,406885,18030C0\n1784,4068B8,1E3F21\n1785,4068E9,1802DA0\n1786,40691C,1E36E1\n1787,406963,1E3641\n1788,406996,1E4040\n1789,4069C7,1802DA0\n1790,4069FA,DE3621\n1791,406A2B,1E4881\n1792,406B7A,1E3A81\n1793,406CC7,1E4961\n1794,406D10,1802EE1\n1795,406D59,1802E00\n1796,406DA6,18030A0\n1797,408A3D,1E4061\n1798,408AAC,1E3A60\n1799,408B29,1E3500\n1800,408B98,1E3960\n1801,408C0B,1E3B61\n1802,408DBC,1E3DE0\n1803,408E05,1E37A1\n1804,408E4C,1E3BC1\n1805,408EA9,1E3461\n1806,408F64,1E35E1\n1807,40903D,1E3740\n1808,4091BC,1E35C0\n1809,409203,1E3B01\n1810,409C1A,BE3280\n1811,409D47,BE3261\n1812,4119D6,1FE3440\n1813,411A1D,1FE3F60\n1814,411A66,1FE3840\n1815,41A6EB,BE3341\n1816,41A732,BE3541\n1817,41A779,BE33E1\n1818,41A910,BE3140\n1819,41AA3B,BE3261\n1820,41ABD2,BE3341\n1821,433B13,1FE3681\n1822,433B5A,1FE4040\n1823,433BA9,1FE4661\n1824,433BF0,1FE3D20\n1825,433C21,1FE40C1\n1826,433C60,1FE3840\n1827,433C91,1FE33E1\n1828,433CC4,7E3F21\n1829,433CF5,1FE3EE0\n1830,433D32,1FE4860\n1831,433D63,DE3C81\n1832,433DA2,1FE4121\n1833,433DD3,1FE44E1\n1834,436BB6,5E34A0\n1835,436D59,1802F80\n1836,436D8C,5E3421\n1837,436DBD,5E26E1\n1838,436DF0,5E3540\n1839,436E21,18030E1\n1840,436E54,DE3621\n1841,436E91,1802EE1\n1842,436EC4,5E3DA0\n1843,436EF5,1E39C0\n1844,436F28,1802F01\n1845,436F61,5E37E1\n1846,436F94,1803120\n1847,4370A3,1E3801\n1848,4371DE,1E3820\n1849,437221,1E3740\n1850,43726A,1E3840\n1851,4372B3,1802E41\n1852,437330,1802D00\n1853,437361,1E3BE0\n1854,437458,1E3820\n1855,437495,1E3C41\n1856,4374D4,1E3660\n1857,43751B,1E3960\n1858,43754E,1E3941\n1859,43757F,1802D41\n1860,4375B2,1E42C0\n1861,4375E3,1E4460\n1862,437632,DE3780\n1863,437663,1E33C0\n1864,4376DC,1E3740\n1865,43774F,1E3AC0\n1866,437782,1802B81\n1867,4377B3,DE3D61\n1868,4377F4,1E3621\n1869,43783B,1802F61\n1870,4378A4,1E3BC1\n1871,4378ED,1802F40\n1872,437954,1E3C41\n1873,437AA1,1E40C1\n1874,437BA8,18030C0\n1875,43997F,1E37E0\n1876,439A4E,1E3341\n1877,439A83,1E34E0\n1878,439B34,1E3C21\n1879,439BAB,1E3581\n1880,439BF4,1E4301\n1881,439CE5,1E3CE1\n1882,43AAE0,5E3121\n1883,43AB2B,BE3541\n1884,43ACCC,BE3321\n1885,44281F,1FE34A1\n1886,442868,1FE3880\n1887,44A541,BE34A1\n1888,44A6DE,BE3180\n1889,44A82F,BE3420\n1890,46488E,1FE37A1\n1891,4648D7,1FE4841\n1892,464922,1FE4D21\n1893,46495F,1FE3440\n1894,464996,1FE39E1\n1895,4649C7,DE3740\n1896,4649FA,1FE4B00\n1897,464A2B,7E3861\n1898,464A5E,1FE3381\n1899,464A8F,7E3CE1\n1900,464AC2,1FE5081\n1901,466CBB,1802FA1\n1902,46768E,5E2FE1\n1903,4677DF,5E3281\n1904,46782E,1803041\n1905,467FE7,1E36A0\n1906,46801A,1E3C81\n1907,46804B,DE43E0\n1908,46809A,1802E21\n1909,4680CB,1E4361\n1910,4680FE,1802FA1\n1911,46813D,1E3E40\n1912,468170,1802D00\n1913,4681A1,1E3E80\n1914,4681EA,1E3B01\n1915,468235,1E39E1\n1916,468268,1E3541\n1917,4682A1,1E36C0\n1918,4682D4,DE33A0\n1919,468313,1E3820\n1920,46834E,1E39E1\n1921,468395,1E4B60\n1922,468442,1E3B40\n1923,46847D,1E34C1\n1924,4684B0,1E3C81\n1925,4684E7,1E3500\n1926,468532,DE3820\n1927,468563,1802C40\n1928,468596,DE3321\n1929,4685E5,1802EA0\n1930,468618,1E4841\n1931,46868F,1E42E1\n1932,4686D6,18030A0\n1933,46A873,1E3780\n1934,46A8EA,1E3420\n1935,46AAA1,1E35C0\n1936,46AB1C,1E3621\n1937,46AC77,1E3840\n1938,46AE80,1E36A0\n1939,46B8E1,BE3621\n1940,47C082,BE3401\n1941,47C0D3,BE32A1\n1942,47C1C4,BE3360\n1943,47C31B,BE3461\n1944,4955AC,1FE3900\n1945,4955F3,1FE4301\n1946,495626,1FE3541\n1947,495661,1FE38E0\n1948,4956A0,1FE3B80\n1949,4956E9,1FE4D21\n1950,49571C,1FE3CA0\n1951,495765,DE3201\n1952,495798,1FE4EC0\n1953,4957C9,7E3660\n1954,4957FC,1FE3880\n1955,49582D,7E3621\n1956,495860,1FE4040\n1957,495891,7E3921\n1958,498396,1802BE1\n1959,4984BD,5E33E0\n1960,498624,1802DE1\n1961,498681,1802881\n1962,4986CE,1E4781\n1963,498717,DE31C1\n1964,498968,1802CA1\n1965,4989B3,1E3840\n1966,498AE0,1E3CE1\n1967,498B87,1803060\n1968,498BD4,1E36C0\n1969,498C1B,1E3740\n1970,498C5A,1E39E1\n1971,498C8B,DE3621\n1972,498CE8,1803541\n1973,498D19,1E45C1\n1974,498D74,1E3681\n1975,498DB5,1802DC0\n1976,498E02,1E3D20\n1977,498E45,1E4320\n1978,498E8E,1E3A60\n1979,498ED7,1E38E0\n1980,498F3E,1E35A0\n1981,498F9B,1E3541\n1982,498FDC,1E3D01\n1983,49900D,1803641\n1984,499040,1E3CC0\n1985,499071,1803541\n1986,4990A4,DE3761\n1987,4990F3,1803440\n1988,499126,1E3F41\n1989,499167,1E3D40\n1990,49919A,1E4001\n1991,4991CB,1802DA0\n1992,4991FE,1E3A21\n1993,499267,1E3761\n1994,4992B0,18039A0\n1995,4992E1,1E39A0\n1996,4993D8,1802F20\n1997,4994BD,1E37A1\n1998,49950E,1803220\n1999,499717,1802C61\n2000,499AE4,1803000\n2001,49B4AD,1E3F00\n2002,49B52E,1E39C0\n2003,49B5EB,1E3A00\n2004,49B632,1E3DA1\n2005,49B663,1E3500\n2006,49B6AC,DE3A00\n2007,49B6DD,1E3261\n2008,49B75C,1E35A0\n2009,49B7AB,1E39C0\n2010,49B7F8,1E3900\n2011,49B829,1E3761\n2012,49B9D8,1E37E0\n2013,49C7B5,BE3801\n2014,4A425A,1FE3B61\n2015,4A42CD,1FE37E0\n2016,4A4300,1FE3641\n2017,4A4331,DE3701\n2018,4A4364,1FE3521\n2019,4A43B3,1FE3900\n2020,4AC596,BE2C40\n2021,4AC629,BE3500\n2022,4AC8F8,BE3120\n2023,4ACB73,BE3300\n2024,4C622A,1FE34A1\n2025,4C6271,1FE4441\n2026,4C62BA,1FE3C21\n2027,4C62EB,1FE3541\n2028,4C6332,1FE3B80\n2029,4C6377,1FE4001\n2030,4C63AA,1FE3440\n2031,4C63ED,1FE3C00\n2032,4C6420,1FE34A1\n2033,4C6459,1FE3440\n2034,4C6498,1FE38A1\n2035,4C64C9,1FE4721\n2036,4C6504,1FE42E1\n2037,4C6535,DE4A40\n2038,4C656E,1FE3C60\n2039,4C65D7,1FE4460\n2040,4C660A,7E35C0\n2041,4C9141,5E32A0\n2042,4C9188,5E32C0\n2043,4C91FB,5E3001\n2044,4C97C2,1E3DE0\n2045,4C980B,1E3720\n2046,4C986A,1E3880\n2047,4C98B9,1E4121\n2048,4C98FC,1E36C0\n2049,4C9943,1E4340\n2050,4C9A3C,1E33A0\n2051,4C9AC3,1E3560\n2052,4C9AF6,1E3861\n2053,4C9B27,1E3BE0\n2054,4C9B5A,DE36E1\n2055,4C9B8B,1E3E40\n2056,4C9BDE,1E3B80\n2057,4C9C27,1E4EE1\n2058,4C9D30,1E40A1\n2059,4C9DA1,1E3B01\n2060,4C9DD4,1E36C0\n2061,4C9E05,DE3581\n2062,4C9E44,1E39E1\n2063,4C9F9B,1E3A41\n2064,4CA008,1E3E80\n2065,4CBD65,1E48E1\n2066,4CC29E,1E3641\n2067,4CC321,1E39A0\n2068,4CC38E,1E3960\n2069,4CC431,1E3681\n2070,4CC480,DE3300\n2071,4CC4B1,1E3DA1\n2072,4CC4E8,1E3C00\n2073,4CC559,1E36E1\n2074,4CC5E2,1E3A21\n2075,4CC631,1E3DC1\n2076,4CC8EA,1E3840\n2077,4CD459,BE3360\n2078,4CD592,BE3461\n2079,4D5085,1FE39A0\n2080,4D50CE,1FE39C0\n2081,4D5115,1FE3761\n2082,4DD62C,BE3101\n2083,4DD673,BE3681\n2084,4DD6AA,BE3021\n2085,4DD801,BE3500\n2086,4F70B8,1FE3A00\n2087,4F70FF,1FE3CC0\n2088,4F7148,1FE3D20\n2089,4F7185,1FE37A1\n2090,4F71C8,1FE3CE1\n2091,4F71F9,1FE3360\n2092,4F7236,1FE3941\n2093,4F7271,1FE35C0\n2094,4F72A4,1FE3D40\n2095,4F72DF,1FE4700\n2096,4F7312,7E3461\n2097,4F7343,1FE3C00\n2098,4F7376,DE41E1\n2099,4F73AF,1FE44E1\n2100,4F73FA,7E3761\n2101,4FA14B,5E3640\n2102,4FA64A,1E3EA1\n2103,4FA9B7,1E36E1\n2104,4FA9F4,1E37C1\n2105,4FAA3D,1E3480\n2106,4FAA86,1E36A0\n2107,4FAACD,1E37E0\n2108,4FABBC,1E3761\n2109,4FABED,1E3660\n2110,4FAC20,DE37E0\n2111,4FAC51,1E3A60\n2112,4FACBE,1E3861\n2113,4FACF7,1E36E1\n2114,4FAD38,DE33E1\n2115,4FAD69,1E3C00\n2116,4FADB8,1E3801\n2117,4FADE9,1E32E0\n2118,4FAE2C,1E3D61\n2119,4FAE5D,1E36A0\n2120,4FAE90,DE3321\n2121,4FAEFD,1E47E1\n2122,4FAF3C,1E4961\n2123,4FAF83,1E3DE0\n2124,4FAFB6,1E3E80\n2125,4FAFF3,1E39C0\n2126,4FB0E6,1E36C0\n2127,4FB165,1E3BC1\n2128,4FB232,1E35C0\n2129,4FB29B,1E3621\n2130,4FB438,1E3900\n2131,4FCF17,1E4340\n2132,4FD032,1E3761\n2133,4FD079,1E34E0\n2134,4FD0C0,1E4241\n2135,4FD0FD,1E3720\n2136,4FD184,1E3500\n2137,4FD2C3,1E3500\n2138,4FD30C,1E4661\n2139,4FE0E5,BE3261\n2140,4FE120,BE31A1\n2141,4FE15B,BE3300\n2142,4FE190,BE3300\n2143,4FE1C9,BE30C0\n2144,4FE210,DE3EC1\n2145,505E0F,1FE3060\n2146,505E60,1FE37E0\n2147,50E86B,BE3461\n2148,50E914,BE31A1\n2149,50E9E3,BE35C0\n2150,527E42,1FE31E0\n2151,527E9F,1FE3AC0\n2152,527EDA,1FE3261\n2153,527F0D,1FE3541\n2154,527F44,1FE3500\n2155,527F75,DE3C81\n2156,527FA8,1FE36A0\n2157,527FF3,1FE59C0\n2158,528026,7E37A1\n2159,528057,1FE3EE0\n2160,52808A,7E3861\n2161,5280BB,1FE3BA1\n2162,5280EE,DE4A01\n2163,52811F,1FE4620\n2164,528152,7E39C0\n2165,52AAD5,1802E41\n2166,52AC9C,5E32C0\n2167,52ADF7,5E34E1\n2168,52AEB4,5E3200\n2169,52AF07,1802E60\n2170,52AF3A,5E3320\n2171,52AF8D,5E3421\n2172,52B0AA,1802DE1\n2173,52B181,1E3F41\n2174,52B2D4,1E3761\n2175,52B305,1802F80\n2176,52B590,1E3720\n2177,52B5D7,1E35E1\n2178,52B638,1E3401\n2179,52B67F,1E38A1\n2180,52B6C8,1E3761\n2181,52B6F9,1E33A0\n2182,52B74A,1E36C0\n2183,52B791,1E38A1\n2184,52B7DA,1803120\n2185,52B80B,1E3321\n2186,52B852,1802F80\n2187,52B883,1E35C0\n2188,52B8CC,1E3801\n2189,52B90D,1E39C0\n2190,52B940,1E3420\n2191,52B971,1E4100\n2192,52B9BA,1E4260\n2193,52B9EB,1802E21\n2194,52BA1E,1E4040\n2195,52BA4F,18036E1\n2196,52BA82,1E4400\n2197,52BAB3,18035A0\n2198,52BAE6,DE3480\n2199,52BB35,1E4141\n2200,52BB68,1E36E1\n2201,52BBA5,1E35C0\n2202,52BBD8,18031C1\n2203,52BC09,DE3621\n2204,52BC76,1E3DE0\n2205,52BCB7,1E41C0\n2206,52BE1A,1803060\n2207,52C109,1802D60\n2208,52C378,1E3B01\n2209,52C3A9,1802F40\n2210,52C3EA,1803220\n2211,52DC93,1E3761\n2212,52DCF0,1E3FE1\n2213,52DDE1,1E3541\n2214,52DEC6,1E3681\n2215,52DF25,1E3D40\n2216,52DFE4,1E3B01\n2217,52E0A7,1E3D20\n2218,52EF98,BE3621\n2219,52F237,5E3260\n2220,536B44,1FE34C1\n2221,53ECC5,BE37C1\n2222,53ED0C,BE3240\n2223,558BCB,1FE3A81\n2224,558C16,1FE3BA1\n2225,558C47,1FE4040\n2226,558C90,1FE4920\n2227,558CC1,1FE3341\n2228,558D00,1FE35A0\n2229,558D33,1FE36C0\n2230,558D6C,1FE37A1\n2231,558DD9,1FE3621\n2232,558E26,7E3AA0\n2233,558E57,1FE40C1\n2234,558E8A,DE4001\n2235,558EBB,7E3401\n2236,558EF4,1FE5000\n2237,55B63D,1802E21\n2238,55BB22,5E33E0\n2239,55BB7D,5E3841\n2240,55BC4C,1E37C1\n2241,55BC7D,5E34C0\n2242,55BE12,1E37C1\n2243,55C131,1E3521\n2244,55C2AC,1E3701\n2245,55C2F3,1E34C1\n2246,55C33A,1E3740\n2247,55C37B,1E3960\n2248,55C3C4,1E3900\n2249,55C3F5,1E3740\n2250,55C432,1E3C60\n2251,55C463,DE35E1\n2252,55C496,1E42A0\n2253,55C4C7,DE3900\n2254,55C4FA,1E3E80\n2255,55C541,1E3BA1\n2256,55C5AC,1E36E1\n2257,55C5DD,1E3621\n2258,55C654,1E3F21\n2259,55C693,1E3701\n2260,55C6DC,1E3D01\n2261,55C70D,1E3A60\n2262,55C748,1E3560\n2263,55C779,1803280\n2264,55C7C4,1802C80\n2265,55C7F5,1E4CE0\n2266,55C83E,DE38A1\n2267,55C86F,1803101\n2268,55C8A2,1E3981\n2269,55C929,1E3E40\n2270,55C96A,1E3FA0\n2271,55C99B,1802E00\n2272,55C9CE,1E4F01\n2273,55CA3B,1E3AA0\n2274,55CAE6,1E36A0\n2275,55CB55,1E3E20\n2276,55E766,1E36A0\n2277,55E949,1E3681\n2278,55EABC,1E3D61\n2279,55EAED,1E3CC0\n2280,55EF02,1E3A60\n2281,55FE4F,BE3240\n2282,55FEC6,BE3880\n2283,567923,1FE37A1\n2284,56FB86,BE36C0\n2285,56FCC3,BE3321\n2286,56FD3C,BE3021\n2287,56FE01,BE3280\n2288,56FF7C,BE3161\n2289,57020D,BE3180\n2290,5897A6,1FE3381\n2291,5897ED,1FE3660\n2292,589836,1FE3CA0\n2293,589885,1FE49C1\n2294,5898CE,1FE4601\n2295,589901,1FE3541\n2296,58994A,1FE42A0\n2297,58997B,1FE3A00\n2298,5899BE,1FE3840\n2299,5899EF,1FE3600\n2300,589A22,7E3681\n2301,589A53,1FE3B40\n2302,589A86,DE3BC1\n2303,589AB7,1FE3780\n2304,589AEA,7E3A81\n2305,589B1B,1FE4100\n2306,589B58,1FE4B60\n2307,589B89,1FE4800\n2308,589BBC,DE3A81\n2309,589C23,1FE4741\n2310,58C72E,5E3121\n2311,58C9D1,5E32E1\n2312,58CA20,1E3861\n2313,58CAD3,5E33E0\n2314,58CF2A,1E37C1\n2315,58CFE3,1E3801\n2316,58D02A,1E39A0\n2317,58D071,1E3EA1\n2318,58D0CE,1E3560\n2319,58D0FF,1E3480\n2320,58D270,1E36A0\n2321,58D2B7,1E44E1\n2322,58D2F8,1E3600\n2323,58D361,1E3B20\n2324,58D3A2,1E3801\n2325,58D40D,1E36C0\n2326,58D48E,1E3500\n2327,58D4F5,1E2441\n2328,58D578,1E3921\n2329,58D61D,1E45A1\n2330,58F67E,1E4920\n2331,58F6F1,1E3780\n2332,58F8AC,1E3720\n2333,58F8F5,1E42A0\n2334,58F940,1E3440\n2335,58F993,1E3A00\n2336,58F9DA,1E3701\n2337,58FA21,1E3960\n2338,58FCC6,1E38A1\n2339,58FD5F,1E3E40\n2340,590A80,BE3261\n2341,5A0E95,BE3560\n2342,5A1152,BE2EC0\n2343,5A1189,BE3120\n2344,5BA6A2,1FE3120\n2345,5BA717,1FE3180\n2346,5BA750,1FE35E1\n2347,5BA78F,1FE3A81\n2348,5BA7C2,1FE3521\n2349,5BA7F3,7E3681\n2350,5BA826,1FE44A0\n2351,5BA857,DE3FA0\n2352,5BA88A,1FE43A1\n2353,5BA8BB,7E34A1\n2354,5BA8F4,1FE3CE1\n2355,5BA929,1FE4860\n2356,5BA95C,DE3E80\n2357,5BD36D,5E35E0\n2358,5BD418,5E33A1\n2359,5BDA39,1E37A1\n2360,5BDCAC,1E37C1\n2361,5BDE03,1E3F21\n2362,5BDE46,1E4200\n2363,5BDE77,1E3660\n2364,5BDED4,1E3840\n2365,5BDF05,1E4241\n2366,5BDF80,1E49E0\n2367,5BDFB1,1E33A0\n2368,5BDFE4,1E3A00\n2369,5BE015,1E38E0\n2370,5BE072,1E4040\n2371,5BE0B7,1E3EC1\n2372,5BE0FA,1E39A0\n2373,5BE15F,1E3960\n2374,5BE1C6,1E35C0\n2375,5BE213,1E4800\n2376,5BE25C,1E3FE1\n2377,5BE2B9,1E30A0\n2378,5BE302,1E4CA1\n2379,5BE333,1E3AA0\n2380,5BE36C,1E3D40\n2381,5BE39D,DE3E80\n2382,5BE3D0,1802E81\n2383,5BE401,1E3621\n2384,5BE434,DE3720\n2385,5BE465,1E3740\n2386,5BE592,1E3900\n2387,5BE847,1E4F40\n2388,5C046E,1E35E1\n2389,5C04B5,DE3261\n2390,5C0584,1E39C0\n2391,5C05C5,1E3560\n2392,5C05FA,1E3761\n2393,5C062B,DE39C0\n2394,5C065E,1E3801\n2395,5C0AE7,1E37E0\n2396,5C187A,BE3261\n2397,5D12E7,BE3440\n2398,5D1442,BE3600\n2399,5D15A1,BE3381\n2400,5D15EA,BE33E1\n2401,5D16DB,BE34C1\n2402,5D183C,BE2FC1\n2403,5EB31F,1FE3581\n2404,5EB352,1FE3240\n2405,5EB39B,1FE3AE1\n2406,5EB3E2,1FE34C1\n2407,5EB429,1FE3B40\n2408,5EB460,1FE34E0\n2409,5EB499,1FE3240\n2410,5EB4E2,1FE4160\n2411,5EB513,1FE3660\n2412,5EB554,1FE3EE0\n2413,5EB585,1FE3641\n2414,5EB5B8,7E3761\n2415,5EB5E9,1FE39A0\n2416,5EB61C,DE4061\n2417,5EB64D,1FE3A21\n2418,5EB680,7E3381\n2419,5EB6B1,1FE43C1\n2420,5EE120,5E3141\n2421,5EE151,1802FC1\n2422,5EE1E4,5E33E0\n2423,5EE22B,5E3400\n2424,5EE272,1E36A0\n2425,5EE593,1E3A21\n2426,5EE5DA,1E36A0\n2427,5EE641,1E3A81\n2428,5EE6F2,1E3C21\n2429,5EE739,1E3560\n2430,5EE782,18032C1\n2431,5EE7B3,1E4181\n2432,5EE7FC,1802F61\n2433,5EE82D,1E4100\n2434,5EE860,1E41A0\n2435,5EE8AD,1E49E0\n2436,5EE8E0,1802D60\n2437,5EE911,1E4661\n2438,5EE944,1E3521\n2439,5EE975,1802D41\n2440,5EE9A8,DE3C60\n2441,5EE9D9,1E4001\n2442,5EEA22,1E3C00\n2443,5EEA53,1E3C00\n2444,5EEA90,1E3C60\n2445,5EEAC1,DE3B61\n2446,5EEB3C,1E3420\n2447,5EEB85,1E3CE1\n2448,5EEBB8,1E3A60\n2449,5EEC21,1E3880\n2450,5EEC54,1E3660\n2451,5EEC8F,1E39E1\n2452,5EECC2,1E36C0\n2453,5EECF3,1802E21\n2454,5EED42,1802BE1\n2455,5EED73,1E4441\n2456,5EEDB4,1E3CE1\n2457,5F189F,1E3BA1\n2458,5F190C,1E3840\n2459,5F199B,1E35A0\n2460,5F1A22,1E3560\n2461,5F1AC5,1E3701\n2462,5F1E36,1E3A81\n2463,5F2633,BE3761\n2464,5FA16C,1FE3B01\n2465,602B33,BE32A1\n2466,602C64,BE3360\n2467,602E0F,BE32E0\n2468,602E4A,BE3541\n2469,61C0ED,1FE3A00\n2470,61C136,1FE5180\n2471,61C179,1FE38C1\n2472,61C1C8,1FE54A1\n2473,61C1F9,1FE3761\n2474,61C242,1FE4320\n2475,61C273,1FE3C81\n2476,61C2B0,1FE3C00\n2477,61C2E1,1FE3641\n2478,61C31A,1FE3EE0\n2479,61C34F,1FE4A40\n2480,61C382,7E3560\n2481,61C3B3,1FE40A1\n2482,61C3E6,DE4B81\n2483,61C417,1FE3600\n2484,61E640,1802DE1\n2485,61E68D,1802DE1\n2486,61EC56,1802E21\n2487,61EE07,1802DA0\n2488,61EE4E,5E32E1\n2489,61EEAB,5E3A40\n2490,61EF2C,1803021\n2491,61F269,1802FE0\n2492,61F2B4,1E41E1\n2493,61F56B,18024C0\n2494,61F62C,1E35C0\n2495,61F6D1,1802EE1\n2496,61F7BE,1802F80\n2497,61F801,1E3CE1\n2498,61F93C,1E3CA0\n2499,61F983,1E37A1\n2500,61F9C6,1E3BE0\n2501,61F9F7,1E3761\n2502,61FA40,1E3440\n2503,61FA79,1E3CA0\n2504,61FABC,1E3720\n2505,61FAED,1802F01\n2506,61FB20,1E3960\n2507,61FB69,1E45A1\n2508,61FB9C,1802F20\n2509,61FBCD,1E41E1\n2510,61FC00,1E38C1\n2511,61FC3F,1E34E0\n2512,61FC72,DE36E1\n2513,61FCA3,1E33E1\n2514,61FCE6,1E4340\n2515,61FD17,1802EA0\n2516,61FD4A,1E3CA0\n2517,61FD7B,1802EA0\n2518,61FDAE,DE3541\n2519,61FDDF,1E43C1\n2520,61FE64,1E38C1\n2521,61FEAB,1E4481\n2522,61FF16,1E4980\n2523,61FFB9,1E3E40\n2524,62002A,1E3EC1\n2525,6203AF,1802D81\n2526,621EB4,1E4520\n2527,621F3F,1E3A00\n2528,621FC2,1E3861\n2529,622103,1E3621\n2530,622194,1E3A00\n2531,622343,1E34C1\n2532,622404,1E3761\n2533,62244B,1E3CC0\n2534,623282,BE3701\n2535,63362B,BE33A0\n2536,6338F0,BE33C0\n2537,64CEAD,1FE3660\n2538,64CEE0,1FE37C1\n2539,64CF29,1FE43E0\n2540,64CF5C,1FE37E0\n2541,64CF9D,1FE3740\n2542,64CFD0,1FE3480\n2543,64D001,7E36A0\n2544,64D034,1FE3B40\n2545,64D065,DE3D40\n2546,64D098,1FE4561\n2547,64D0CF,1FE3440\n2548,64FCD2,5E34C0\n2549,65066F,1E3820\n2550,650998,1E3A81\n2551,650B59,1E3B01\n2552,650C48,1E38C1\n2553,650C79,1E38E0\n2554,650CF0,1E39C0\n2555,650D3F,1E4901\n2556,650D8C,1E3641\n2557,650DD3,1E3A60\n2558,650E30,1E3F60\n2559,650EB7,1E3BE0\n2560,650F00,1E38A1\n2561,650F31,1E4AC1\n2562,650F68,1E36C0\n2563,650F99,DE3DE0\n2564,650FCC,1E3941\n2565,651013,1E43A1\n2566,651052,1E3900\n2567,651083,1E3960\n2568,6510CC,DE39E1\n2569,6510FD,1E3D80\n2570,65116C,1E4361\n2571,65141F,1E4881\n2572,65149E,1E3DE0\n2573,651CD7,1E48C0\n2574,65214C,1E42A0\n2575,65230D,1E4020\n2576,652452,1E3960\n2577,65258B,1E3CC0\n2578,6525F4,1E2CE0\n2579,65269B,1E3660\n2580,6526E6,1E3A81\n2581,652717,1E4040\n2582,652750,1E3500\n2583,652781,DE36C0\n2584,6527D2,1E36E1\n2585,652803,1E39C0\n2586,65286E,1E4460\n2587,65289F,DE3FC0\n2588,6528E2,1E3681\n2589,652913,1E3DA1\n2590,65295C,1E40E0\n2591,6529A5,1E3B61\n2592,6529EE,1E3941\n2593,652A5B,1E3740\n2594,652AEA,1E3681\n2595,652B31,1E34E0\n2596,652B78,1E36A0\n2597,652BB9,1E3BC1\n2598,652BFA,1E3C21\n2599,652DC1,1E4100\n2600,652DF4,1E36A0\n2601,652EED,1E3641\n2602,65317E,1E3A41\n2603,654183,BE3820\n2604,6543F6,5E2981\n2605,65BB23,1FE3B01\n2606,65BB6C,1FE3521\n2607,65BBB3,1FE3C00\n2608,65BBFE,1FE30E1\n2609,6647FB,BE34A1\n2610,66495A,BE32A1\n2611,664BED,BE36C0\n2612,664D54,BE2FC1\n2613,664D97,BE3280\n2614,67D9A6,1FE30C0\n2615,67D9ED,1FE3500\n2616,67DA4A,1FE3740\n2617,67DA91,1FE4260\n2618,67DADC,1FE4281\n2619,67DB25,1FE3DC1\n2620,67DB68,1FE3300\n2621,67DBB1,1FE4241\n2622,67DBF8,1FE4F40\n2623,67DC43,1FE4800\n2624,67DC78,1FE3780\n2625,67DCC3,1FE3A21\n2626,67DCF6,1FE3541\n2627,67DD31,1FE3960\n2628,67DD9C,1FE34E0\n2629,67DDDF,7E3341\n2630,67DE12,1FE50C0\n2631,67DE43,7E38A1\n2632,67DE76,1FE53E1\n2633,67DEAD,1FE4700\n2634,67DEE0,DE36A0\n2635,67DF17,1FE4F40\n2636,680D34,5E34E1\n2637,680F3D,1E3720\n2638,680F86,1E44A0\n2639,681091,1E3AE1\n2640,6810DA,1E3681\n2641,68123B,1E3AA0\n2642,681284,1E33C0\n2643,681347,1E3E01\n2644,681390,1803140\n2645,6813C1,1E44A0\n2646,6813FE,1E32E0\n2647,68142F,DE32C1\n2648,681462,1802E60\n2649,681493,1E38A1\n2650,6814CE,1E40A1\n2651,68150F,1E3A41\n2652,681542,DE3440\n2653,681573,1E36E1\n2654,6815A6,DE3921\n2655,6815D7,1E44E1\n2656,681620,1802F80\n2657,681651,1E3B80\n2658,681698,DE3521\n2659,6816C9,1E3461\n2660,681710,1802D81\n2661,681741,1E38C1\n2662,6817C2,1E3DE0\n2663,681871,1E36E1\n2664,6818BA,1802F61\n2665,681905,1802FC1\n2666,6819C6,1E46E0\n2667,681A0F,1803101\n2668,681A42,1E39A0\n2669,681A89,DE3701\n2670,681D38,1802DE1\n2671,6839C9,1E3600\n2672,683AF8,1E32C1\n2673,683B2F,1E3560\n2674,683B68,1E36A0\n2675,683B99,DE36C0\n2676,683CD2,1E3820\n2677,683D19,1E37E0\n2678,683D64,1E31E0\n2679,683DAB,1E4460\n2680,683DFE,1E3A41\n2681,683E57,1E3500\n2682,683EB0,1E37E0\n2683,684CD5,BE3401\n2684,684D10,BE3180\n2685,684D49,BE31A1\n2686,684D92,BE3381\n2687,684DC7,BE3461\n2688,684E0A,DE35A0\n2689,69537D,BE3300\n2690,695462,BE32E0\n2691,6AE6D7,1FE38A1\n2692,6AE720,1FE3780\n2693,6AE76F,1FE3E40\n2694,6AE7CC,1FE3681\n2695,6AE813,1FE3740\n2696,6AE85A,1FE4121\n2697,6AE8A1,1FE35C0\n2698,6AE8EA,1FE3D20\n2699,6AE939,1FE3F81\n2700,6AE988,1FE4901\n2701,6AE9B9,1FE37C1\n2702,6AE9F8,1FE3401\n2703,6AEA29,1FE31C1\n2704,6AEA5C,DE3960\n2705,6AEA8D,1FE3641\n2706,6AEAC8,1FE38E0\n2707,6AEAFD,1FE38E0\n2708,6AEB6A,1FE4421\n2709,6AEB9B,7E3761\n2710,6AEBD6,1FE4BC0\n2711,6B1787,5E35C1\n2712,6B185A,1802F40\n2713,6B188B,5E3DA0\n2714,6B1E36,1E34E0\n2715,6B1F21,1E4721\n2716,6B1F54,1803261\n2717,6B2109,1E3A00\n2718,6B215A,1E3F41\n2719,6B2193,1E36C0\n2720,6B21C6,DE2F01\n2721,6B21F7,1E4421\n2722,6B2246,1802DC0\n2723,6B2287,1E3B40\n2724,6B22D0,1803081\n2725,6B2301,1E3E01\n2726,6B2334,1803420\n2727,6B2365,1E3880\n2728,6B23DA,1E3660\n2729,6B241B,1E3880\n2730,6B244E,1E3840\n2731,6B247F,1802E81\n2732,6B24B2,DE33A0\n2733,6B24E3,1E3761\n2734,6B259E,1E3461\n2735,6B25CF,1E3960\n2736,6B260A,1E3A00\n2737,6B2645,1E38E0\n2738,6B2678,1802EA0\n2739,6B26A9,1E38A1\n2740,6B26DC,1802C61\n2741,6B270D,DE3941\n2742,6B2740,1802E21\n2743,6B2771,1E4640\n2744,6B27A4,1802B81\n2745,6B27D5,1E38C1\n2746,6B280E,1E4100\n2747,6B283F,1802F01\n2748,6B2872,DE3A81\n2749,6B28DF,1E3FC0\n2750,6B2928,18031A1\n2751,6B4B2B,1E3560\n2752,6B4B90,1E2340\n2753,6B4C45,1E3BA1\n2754,6B4D96,1E34A1\n2755,6B5BC5,BE3161\n2756,6BC248,7E2DA0\n2757,6BD73F,1FE3541\n2758,6BD79C,1FE3381\n2759,6C5E7D,BE2A01\n2760,6C5F38,BE3521\n2761,6C60D3,BE31C1\n2762,6C622E,BE3321\n2763,6C6389,BE33A0\n2764,6C63D4,BE36A0\n2765,6C64CB,BE33E1\n2766,6DF6A8,1FE3541\n2767,6DF6EF,1FE3FA0\n2768,6DF722,1FE3180\n2769,6DF76D,1FE4841\n2770,6DF7A0,1FE36E1\n2771,6DF7DB,1FE4721\n2772,6DF80E,1FE3960\n2773,6DF849,1FE3820\n2774,6DF880,1FE3C41\n2775,6DF8B3,1FE3C21\n2776,6DF8E6,7E3621\n2777,6DF917,1FE4741\n2778,6DF94A,DE3F41\n2779,6DF97B,1FE4BE1\n2780,6DF9AE,7E34A1\n2781,6E1EC3,1802B00\n2782,6E20CC,1802DC0\n2783,6E2431,1802EE1\n2784,6E265C,5E3741\n2785,6E26A5,1802C40\n2786,6E26EA,5E3741\n2787,6E271B,1802E41\n2788,6E2776,1802D41\n2789,6E29E3,1E3AA0\n2790,6E2A2E,1E43A1\n2791,6E2B67,1E36C0\n2792,6E2BB0,1E3F41\n2793,6E2C5B,1E36E1\n2794,6E2D58,1802EE1\n2795,6E2F1B,1E37C1\n2796,6E2F4E,1E3CE1\n2797,6E2F7F,DE33C0\n2798,6E2FB2,1E3A41\n2799,6E2FE3,1E39E1\n2800,6E302A,1E4D21\n2801,6E3073,DE34C1\n2802,6E30A6,1E3BC1\n2803,6E313F,1E36A0\n2804,6E3182,1E34C1\n2805,6E31CB,DE3621\n2806,6E31FE,1E3AE1\n2807,6E3295,1E3C00\n2808,6E32C8,1E4400\n2809,6E3307,1E3C41\n2810,6E3456,1E4160\n2811,6E36F5,1E44A0\n2812,6E56AE,1E3B80\n2813,6E56DF,1E3621\n2814,6E5712,DE36A0\n2815,6E5751,1E33E1\n2816,6E57D8,1E3600\n2817,6E5901,1E36A0\n2818,6E594A,1E37C1\n2819,6E5991,1E3880\n2820,6E59DA,1E3801\n2821,6E5A21,1E35A0\n2822,6E6802,BE3381\n2823,6E6875,BE33E1\n2824,6E6BF6,5E34C0\n2825,6EE3DD,1FE3780\n2826,6EE426,1FE40E0\n2827,6EE46F,1FE4F20\n2828,6EE4CC,1FE32C1\n2829,6EE527,1FE3161\n2830,6EE576,1FE3900\n2831,6F6F69,BE3420\n2832,6F6FD6,BE36C0\n2833,6F710D,BE3440\n2834,6F7282,BE32C1\n2835,6F73E1,BE31E0\n2836,6F7502,BE3280\n2837,7104A1,1FE37A1\n2838,71050E,1FE3900\n2839,710559,DE3341\n2840,71058C,1FE3880\n2841,7105D5,1FE4BA0\n2842,710608,1FE3840\n2843,710645,1FE46E0\n2844,710678,7E3DC1\n2845,7106A9,1FE46E0\n2846,7106DC,DE39E1\n2847,71070D,1FE3CA0\n2848,71300A,1802F80\n2849,713055,1802F61\n2850,7132A6,5E32C0\n2851,7134ED,1803220\n2852,713836,1E34E0\n2853,7138E1,1E3AA0\n2854,71392C,1802D60\n2855,713BBD,1802D21\n2856,713BF0,1E3941\n2857,713C6B,1E3720\n2858,713CEE,1E39A0\n2859,713D1F,1803041\n2860,713D52,1E34C1\n2861,713D99,1E48A0\n2862,713DCC,1E35A0\n2863,713DFD,1E3420\n2864,713E30,1802CE0\n2865,713E61,DE3B01\n2866,713E94,1E4181\n2867,713EC5,1E4040\n2868,713EF8,1802DC0\n2869,713F29,1E3740\n2870,713F6A,1E4400\n2871,713FAB,1E3AC0\n2872,713FEC,1E3740\n2873,71401D,1803021\n2874,714050,1E3900\n2875,714087,1E3461\n2876,7140C6,1E3AE1\n2877,7140F7,DE3E61\n2878,714170,1E3740\n2879,71430B,1E3621\n2880,714412,1E40C1\n2881,7145A3,1E5081\n2882,7145EA,1802E81\n2883,716391,1E3840\n2884,716416,1E3C41\n2885,71645F,1E3521\n2886,716492,1E34C1\n2887,716543,1E3861\n2888,7165C6,1E3600\n2889,716601,1E3720\n2890,71677C,1E3B61\n2891,717589,BE36A0\n2892,717600,BE33C0\n2893,717631,BE2841\n2894,71766C,BE33C0\n2895,7176A3,BE34A1\n2896,7176D6,BE3521\n2897,717707,DE3D01\n2898,71F06E,1FE36C0\n2899,71F0E1,1FE3280\n2900,71F128,1FE3300\n2901,71F16F,1FE34E0\n2902,727962,BE3300\n2903,727AB5,BE32A1\n2904,727C12,BE3341\n2905,727D55,BE3341\n2906,727EB2,BE3681\n2907,741073,1FE3201\n2908,7410BC,1FE3B80\n2909,741103,1FE32C1\n2910,74114C,1FE3921\n2911,741191,1FE3F00\n2912,7411C4,1FE3500\n2913,741203,1FE4441\n2914,741236,1FE3E61\n2915,74126F,1FE4241\n2916,7412A2,1FE3761\n2917,7412D3,DE4121\n2918,741306,1FE3D61\n2919,741337,7E3921\n2920,74136A,1FE52C1\n2921,7414C7,7E3AE1\n2922,743712,1802FE0\n2923,74375D,1802E41\n2924,743E42,5E35E0\n2925,744049,5E33C1\n2926,74407C,1802E00\n2927,7440F3,5E3B60\n2928,744126,1802FA1\n2929,744157,DE3820\n2930,7442A8,1802E60\n2931,744713,1802F01\n2932,744762,1E3FA0\n2933,74490B,1802C61\n2934,744966,1E3820\n2935,7449B5,1E4040\n2936,7449FE,1802D21\n2937,744A2F,1E3360\n2938,744B0C,1E3900\n2939,744B3D,1E3600\n2940,744BB6,1E3581\n2941,744BED,1E37E0\n2942,744C88,1E3EE0\n2943,744CB9,1E3B20\n2944,744D84,1E3900\n2945,744E6D,1E49C1\n2946,744EEE,1E3820\n2947,744F1F,1E3560\n2948,744F60,1E43E0\n2949,744FA7,18036A0\n2950,74509E,1E4680\n2951,745205,1802F61\n2952,7454F8,1802DE1\n2953,7471D5,1E3621\n2954,747208,1E3B80\n2955,7472C7,1E31A1\n2956,747334,1E35A0\n2957,747509,1E37E0\n2958,74753C,1E37E0\n2959,747585,1E3F41\n2960,7476B4,1E3B01\n2961,748471,BE3541\n2962,74E9FA,7E30C0\n2963,74EA47,7E3500\n2964,74FE54,1FE3820\n2965,758D91,BE3360\n2966,758E68,BE3581\n2967,75904B,BE32A1\n2968,7591F2,BE3140\n2969,759231,BE3220\n2970,759322,BE3261\n2971,771E5D,1FE31E0\n2972,771EA6,1FE3521\n2973,771EEF,1FE4040\n2974,771F22,1FE3120\n2975,771F6D,1FE4001\n2976,771FA2,1FE36A0\n2977,771FDD,1FE3C81\n2978,772010,1FE36A0\n2979,772047,1FE33E1\n2980,772090,DE3341\n2981,7720C1,1FE4E00\n2982,7720F4,7E3720\n2983,772125,DE3B20\n2984,772158,1FE4260\n2985,7721BD,1FE2A61\n2986,774D2A,5E36E0\n2987,774DDD,5E3121\n2988,774E88,5E3061\n2989,774EF1,5E3D60\n2990,77500C,1802F40\n2991,7751E3,1802E81\n2992,77566E,1E3861\n2993,77573D,1E3C00\n2994,775786,1E3701\n2995,775831,1E3A81\n2996,77587A,1802E00\n2997,7758AB,1E36E1\n2998,7758EA,1E3921\n2999,775931,1E36E1\n3000,77596C,1802E81\n3001,77599D,1E4281\n3002,7759FA,1E3AE1\n3003,775A43,1E36C0\n3004,775A88,1E3DC1\n3005,775B0F,1802F01\n3006,775B42,1E37C1\n3007,775BBF,1E3960\n3008,775C66,1E3701\n3009,775CB5,1803161\n3010,775CE8,1E4A40\n3011,775D6B,1E3D80\n3012,775DB6,1802DC0\n3013,775DE7,1E3621\n3014,777A46,1E4E81\n3015,777DAB,1E3EC1\n3016,777DDE,1E43A1\n3017,777EFD,1E3880\n3018,777F30,1E34C1\n3019,777F73,1E3C00\n3020,777FD0,1E3D01\n3021,778019,1E3621\n3022,7780FC,1E34A1\n3023,77813B,1E3801\n3024,77816E,DE31E0\n3025,77819F,1E3541\n3026,77910E,BE36A0\n3027,7894BD,BE32E0\n3028,789622,BE3120\n3029,789799,BE34E0\n3030,789E2C,BE3021\n3031,7A2CFD,1FE3401\n3032,7A2D48,1FE3B80\n3033,7A2D79,1FE37A1\n3034,7A2DB6,1FE3CE1\n3035,7A2DE9,1FE3BE0\n3036,7A2E22,1FE38E0\n3037,7A2E53,7E33E1\n3038,7A2E86,DE3401\n3039,7A2EB7,1FE4340\n3040,7A2EEA,7E3381\n3041,7A2F1B,1FE37E0\n3042,7A55DA,1802DC0\n3043,7A58A7,1802CA1\n3044,7A5954,5E3540\n3045,7A5A8D,5E3441\n3046,7A679C,1E3A81\n3047,7A686F,1E3581\n3048,7A6980,1E3F41\n3049,7A69C7,1E3B40\n3050,7A6A06,1E3A21\n3051,7A6A4F,1E35E1\n3052,7A6A9C,1E43A1\n3053,7A6ACD,1E3761\n3054,7A6B1E,1E3801\n3055,7A6B4F,1802FC1\n3056,7A6B82,1E42A0\n3057,7A6BEB,1E38C1\n3058,7A6C34,1E3840\n3059,7A6C65,1E39A0\n3060,7A6C98,1803060\n3061,7A6CC9,DE3401\n3062,7A6D02,1E3801\n3063,7A6DB3,1E3A81\n3064,7A6F12,1E3C81\n3065,7A7091,1802DE1\n3066,7A799A,1E45C1\n3067,7A8413,1E3921\n3068,7A86CA,1E3880\n3069,7A896D,1E37C1\n3070,7A89C8,1E3E61\n3071,7A8B15,1E38E0\n3072,7A8C34,1E3C81\n3073,7A9EE3,BE33A0\n3074,7B1AC8,1FE3581\n3075,7B9C41,BE3560\n3076,7B9D80,BE37C1\n3077,7B9EBB,BE3900\n3078,7D3974,1FE34C1\n3079,7D39BB,1FE3820\n3080,7D3A04,1FE3B01\n3081,7D3A4B,1FE3401\n3082,7D3A92,1FE3F21\n3083,7D3AC9,1FE34A1\n3084,7D3B0A,1FE3681\n3085,7D3B3B,DE3941\n3086,7D3B6E,1FE35A0\n3087,7D3BA7,1FE3581\n3088,7D3BDA,7E3541\n3089,7D3C0B,1FE38E0\n3090,7D3C3E,7E38E0\n3091,7D3C6F,1FE3E20\n3092,7D3CA2,DE3CA0\n3093,7D3CD3,1FE6041\n3094,7D3D06,7E3D80\n3095,7D66E1,5E33A1\n3096,7D678C,5E3400\n3097,7D6995,1E3A21\n3098,7D6C96,1E3801\n3099,7D6CDD,1E3AE1\n3100,7D6D10,1E38A1\n3101,7D6D87,1E35E1\n3102,7D6DD6,1E4020\n3103,7D6E17,1E34C1\n3104,7D6E54,1E3E01\n3105,7D6E9B,1E3F21\n3106,7D6ECE,1E4A40\n3107,7D6F0F,1E31E0\n3108,7D6F50,1E38A1\n3109,7D6F81,1E3720\n3110,7D6FDE,1E3B01\n3111,7D700F,1E3AA0\n3112,7D7060,1E3E20\n3113,7D7091,1E3900\n3114,7D70EA,1E3660\n3115,7D711B,1E3681\n3116,7D71E4,1E3B01\n3117,7D724F,1E3E40\n3118,7D728E,1E4800\n3119,7D72CF,1E4AE0\n3120,7D7302,1E3C00\n3121,7D7337,1E3981\n3122,7D737A,1E3F41\n3123,7D73AB,1E4160\n3124,7D73E8,1E3B61\n3125,7D7419,DE4481\n3126,7D9AD2,1E45E0\n3127,7D9E77,1E3F60\n3128,7D9EAA,1E3461\n3129,7D9FA1,1E35E1\n3130,7DA04C,1E3861\n3131,7DA0DB,1E3BA1\n3132,7DA124,1E3A21\n3133,7DA177,1E3900\n3134,7DA220,1E3660\n3135,7DACCD,BE3780\n3136,7DAEF4,5E32C0\n3137,7E2771,1FE4540\n3138,7EAFA8,BE3420\n3139,7EAFEF,BE3DA1\n3140,7EB070,BE35E1\n3141,7EB189,BE2BC0\n3142,7EB378,BE3261\n3143,7EB4BF,BE3021\n3144,7EB4FE,BE30E1\n3145,7EB539,BE3321\n3146,7EB5F4,BE3360\n3147,7FE2F5,1E3261\n3148,804612,1FE3420\n3149,804659,1FE4640\n3150,80469A,1FE33A0\n3151,8046CB,1FE32A1\n3152,804704,1FE3CA0\n3153,80474D,1FE5321\n3154,804780,1FE3DC1\n3155,8047B7,1FE3261\n3156,8047EA,DE3EC1\n3157,80481B,1FE3DE0\n3158,804854,1FE3A41\n3159,804889,1FE4620\n3160,8048C0,1FE4160\n3161,8048F1,DE3541\n3162,804924,1FE3C21\n3163,804955,7E3941\n3164,80498E,1FE45A1\n3165,8049BF,7E3420\n3166,806D16,1802C61\n3167,806D61,18030A0\n3168,8070A8,1803041\n3169,8075F5,1802C80\n3170,807628,5E3680\n3171,8078CF,1E3D80\n3172,807A2E,1E37A1\n3173,807B81,1E3840\n3174,807C34,1E3E01\n3175,807C65,1802D60\n3176,807CC2,1E3AE1\n3177,807D09,1E3B01\n3178,807D54,1E35A0\n3179,807D91,1E3FA0\n3180,807DDA,1E4601\n3181,807E5B,1E3681\n3182,807EA4,1E3641\n3183,807EEB,1E4961\n3184,807F1E,1E38A1\n3185,807F4F,1802E81\n3186,807F82,1E3E40\n3187,807FC5,1E38C1\n3188,808004,1E4460\n3189,808045,1E45E0\n3190,808082,DE3161\n3191,8080B3,1E32A1\n3192,8080EE,1E3CA0\n3193,80811F,18034A1\n3194,808152,1E3840\n3195,8081BB,1E3AC0\n3196,8081EE,1E3D61\n3197,808229,1E3981\n3198,80825C,1802DA0\n3199,80828D,1E3B61\n3200,8082F6,18028C0\n3201,808327,1E52A1\n3202,8084BC,1E3861\n3203,808505,1802F01\n3204,80ACE8,1E3541\n3205,80AE0D,1E39E1\n3206,80B826,BE2FC1\n3207,80B949,BE3261\n3208,80BCFE,5E2641\n3209,81BBE3,BE3321\n3210,81BD3E,BE3341\n3211,81BD83,BE32C1\n3212,81BDCA,BE3521\n3213,81BE77,BE3600\n3214,81C3C0,BE3220\n3215,8354ED,1FE3681\n3216,83552E,1FE3941\n3217,83555F,1FE3201\n3218,835592,DE3921\n3219,8355C3,1FE3C41\n3220,83560C,1FE5041\n3221,83563D,1FE38E0\n3222,835670,7E33A0\n3223,8356A1,1FE3921\n3224,8356D4,DE3560\n3225,835705,1FE44E1\n3226,835738,7E3360\n3227,835769,1FE3D01\n3228,837F22,1802D60\n3229,838285,5E37E1\n3230,83832C,5E3421\n3231,838399,5E34E1\n3232,8383CC,DE3341\n3233,8384AB,1E36C0\n3234,8384F4,1802EE1\n3235,838525,DE3900\n3236,838762,1E3A60\n3237,8387D5,1E3C41\n3238,8388BE,1E38C1\n3239,8388EF,1E3A41\n3240,838922,DE3440\n3241,83896B,1E3641\n3242,83899E,1E36C0\n3243,8389E7,1802DC0\n3244,838A1A,1E3B01\n3245,838A4B,1E38E0\n3246,838A7E,1802CE0\n3247,838AAF,1E41C0\n3248,838AE2,1803180\n3249,838B13,1E3AC0\n3250,838B54,1E4860\n3251,838B85,1802DA0\n3252,838BB8,DE39C0\n3253,838BE9,1E4520\n3254,838C28,1E46A1\n3255,838C65,1E37A1\n3256,838C98,1E3B61\n3257,838CC9,DE4061\n3258,838CFC,1E4881\n3259,838D2D,1802E41\n3260,838D60,1E41C0\n3261,838DA3,1E37A1\n3262,838ED6,18030A0\n3263,838F23,1802C40\n3264,838F56,1E3A81\n3265,838FF7,1802BC0\n3266,839222,1802EE1\n3267,83B531,1E3C00\n3268,83B68E,1E37C1\n3269,83B737,1E3BA1\n3270,83B7AC,1E3C81\n3271,83B95F,1E38E0\n3272,83C71C,BE3341\n3273,844239,1FE35A0\n3274,844282,1FE3D01\n3275,8442D1,1FE3581\n3276,844320,1FE39C0\n3277,844365,1FE35C0\n3278,84C82E,BE37E0\n3279,8661EB,1FE3801\n3280,866232,1FE4241\n3281,866279,1FE46C1\n3282,8662BA,1FE4160\n3283,8662EB,1FE33A0\n3284,86631E,1FE3581\n3285,86634F,DE3960\n3286,866382,1FE5DE0\n3287,8663C9,1FE4860\n3288,8663FC,7E33A0\n3289,86642D,1FE4821\n3290,866460,DE3BA1\n3291,866491,1FE53E1\n3292,8664C4,7E36E1\n3293,8664F5,1FE4DA0\n3294,8682F0,1802F20\n3295,868435,1802C40\n3296,8686E8,1802E41\n3297,86904D,1E3A21\n3298,869080,5E3DE1\n3299,8690F5,5E3721\n3300,86913C,DE3CA0\n3301,869185,5E34A0\n3302,869648,1E3720\n3303,8697C7,1E3720\n3304,869810,1E3E01\n3305,869857,1E3C81\n3306,86988A,1E3BC1\n3307,8698BB,1E3840\n3308,8698EE,1E40A1\n3309,869939,DE3BA1\n3310,86996C,1E3861\n3311,8699B1,1E3780\n3312,8699F8,1E37C1\n3313,869A29,1E3401\n3314,869A72,DE3440\n3315,869AA3,1E3A21\n3316,869AEC,1E3AC0\n3317,869B2B,1E3621\n3318,869B5E,1E3DE0\n3319,869B97,1E37A1\n3320,869BDE,DE45C1\n3321,869C0F,1E4B41\n3322,869C42,1E3E80\n3323,869C81,1E3440\n3324,869CEC,1E3B61\n3325,869D2F,1E3A00\n3326,869D62,DE3B01\n3327,869D93,1E3CA0\n3328,869DC6,DE31E0\n3329,869DF7,1E3660\n3330,869E2A,1E35E1\n3331,869E71,1E47C0\n3332,869EA4,DE3541\n3333,869F13,1E3B80\n3334,86AC46,1802D81\n3335,86BD49,1E4400\n3336,86C2C8,1E3C21\n3337,86C45F,1E3660\n3338,86C4A8,1E33C0\n3339,86C4F1,1E3C60\n3340,86C548,1E3D61\n3341,86C5E1,1E3EC1\n3342,86C630,1E3B80\n3343,86C67F,1E37A1\n3344,86C70E,1E3761\n3345,86C757,1E3820\n3346,86C79E,1E3461\n3347,86C7E5,1E3740\n3348,86D350,BE31C1\n3349,874F93,1FE3B61\n3350,87E0B8,BE3081\n3351,87E1CD,BE3201\n3352,87E20A,BE3240\n3353,87E2ED,BE3060\n3354,87E450,BE32A1\n3355,896ECD,1FE3C81\n3356,896F00,1FE3000\n3357,896F3F,1FE34A1\n3358,896F72,DE3341\n3359,896FA3,1FE3F00\n3360,896FE2,1FE4061\n3361,897013,1FE3DC1\n3362,89704E,1FE3341\n3363,89707F,1FE3A41\n3364,8970B2,DE4721\n3365,8970E7,1FE34A1\n3366,8971D2,7E38A1\n3367,89947F,1802FE0\n3368,899590,1802F01\n3369,899B71,5E3221\n3370,899BB0,1E3641\n3371,899BF7,5E3361\n3372,899D78,5E3540\n3373,899E67,1E3560\n3374,89A06C,1E3C21\n3375,89A0BF,1E3801\n3376,89A108,1E3300\n3377,89A141,1E34E0\n3378,89A188,DE3780\n3379,89A1B9,1E4380\n3380,89A232,1E37C1\n3381,89A27B,1E38E0\n3382,89A2C4,1E48A0\n3383,89A2F5,1E3541\n3384,89A352,1E3560\n3385,89A383,1E4340\n3386,89A402,1E3541\n3387,89A449,1E3BE0\n3388,89A47C,1E3A60\n3389,89A4FD,1E35E1\n3390,89A534,1E35A0\n3391,89A57D,DE45A1\n3392,89A5B0,1E4BE1\n3393,89A623,1E39C0\n3394,89A698,1E3621\n3395,89A6DF,DE3081\n3396,89A7E6,1E3EC1\n3397,89A86B,1E3F60\n3398,89BA9A,1802EE1\n3399,89D72B,1E4061\n3400,89D8D8,1E3B80\n3401,89D921,1E3B40\n3402,89D970,1E3941\n3403,89DA85,1E35A0\n3404,89E24A,BE3960\n3405,89E653,5E34A0\n3406,8ADCB4,BE3120\n3407,8ADE3B,BE33E1\n3408,8C7B18,1FE34A1\n3409,8C7B67,1FE4BC0\n3410,8C7BB2,1FE4721\n3411,8C7BFD,1FE3F00\n3412,8C7C44,1FE3F21\n3413,8C7C8D,1FE3C41\n3414,8C7CCE,1FE34A1\n3415,8C7CFF,1FE3641\n3416,8C7D3C,1FE3500\n3417,8C7D79,1FE3621\n3418,8C7DAC,DE3300\n3419,8C7DDD,1FE3981\n3420,8C7E28,1FE4760\n3421,8C7E59,1FE3300\n3422,8C7E8C,7E39C0\n3423,8C7EBD,1FE4260\n3424,8C7EF0,DE34E0\n3425,8C7F21,1FE4F40\n3426,8C7F54,7E3641\n3427,8C9F07,1802DA0\n3428,8CA226,1802E00\n3429,8CA365,1802E81\n3430,8CA72E,1803280\n3431,8CA847,5E36E0\n3432,8CA978,5E3040\n3433,8CA9FF,5E34C0\n3434,8CAA48,5E3721\n3435,8CAA8F,5E3841\n3436,8CADCE,1E36C0\n3437,8CAE3F,1803060\n3438,8CAEDA,1802EC0\n3439,8CB045,1E3500\n3440,8CB08C,1E39E1\n3441,8CB137,1E3660\n3442,8CB188,1E37A1\n3443,8CB24D,1E3941\n3444,8CB280,1E4460\n3445,8CB2C7,1E3BA1\n3446,8CB31E,1E3A60\n3447,8CB34F,1E39C0\n3448,8CB38E,1E3CC0\n3449,8CB3C7,1E3C60\n3450,8CB448,1E38A1\n3451,8CB479,1E36A0\n3452,8CB4BC,1E4800\n3453,8CB4ED,DE43C1\n3454,8CB542,1E3B80\n3455,8CB5B5,1E3941\n3456,8CB5E8,1E38C1\n3457,8CB667,1E39C0\n3458,8CB7FC,1E4841\n3459,8CB869,1E4540\n3460,8CB8D6,1E4421\n3461,8CC14F,1802860\n3462,8CC1CC,1802C61\n3463,8CC5B3,1802E41\n3464,8CC5FC,1202DC0\n3465,8CC7BD,1803021\n3466,8CDE70,1E5A00\n3467,8CE0DB,1E37A1\n3468,8CE23E,1E39E1\n3469,8CE317,1E3660\n3470,8CE38A,1E4421\n3471,8CE3BB,1E43A1\n3472,8CE404,1E3840\n3473,8CE435,1E38C1\n3474,8CE47E,DE3780\n3475,8CE5E5,1E3560\n3476,8CF054,BE3280\n3477,8CF2C9,5E3700\n3478,8D6B16,1FE3541\n3479,8D6B5D,1FE3261\n3480,8D6BA4,1FE38C1\n3481,8D6BF3,1FE3FC0\n3482,8DF176,BE35A0\n3483,8DF357,BE3261\n3484,8DF58A,BE3300\n3485,8DF5C9,BE32A1\n3486,8DF6DC,BE3440\n3487,8F891F,1FE36A0\n3488,8F8968,1FE3500\n3489,8F89AF,1FE3B80\n3490,8F89FA,1FE3E40\n3491,8F8A2B,1FE3C81\n3492,8F8A72,1FE3FE1\n3493,8F8AA7,1FE3261\n3494,8F8AE4,1FE37E0\n3495,8F8B15,1FE34E0\n3496,8F8B48,DE3E80\n3497,8F8B79,1FE3D61\n3498,8F8BB8,1FE3840\n3499,8F8BE9,1FE3CE1\n3500,8F8C1C,7E3440\n3501,8F8C4D,1FE44C0\n3502,8F8C80,DE3F21\n3503,8F8CB1,1FE4B81\n3504,8F8CE4,7E3720\n3505,8F8D15,1FE4BE1\n3506,8F8D48,7E3BA1\n3507,8FA4C5,1802E21\n3508,8FA816,1803021\n3509,8FB76B,5E3260\n3510,8FB7DA,5E30E0\n3511,8FB81F,DE3861\n3512,8FBE58,1E3521\n3513,8FBE9F,1E34A1\n3514,8FBEF0,1E4061\n3515,8FBF91,1E3A21\n3516,8FC01A,1E3401\n3517,8FC04B,1E3D80\n3518,8FC08E,1E3761\n3519,8FC0C9,1E3500\n3520,8FC10C,1E37A1\n3521,8FC13D,1E3AE1\n3522,8FC170,DE3541\n3523,8FC1A1,1E3AE1\n3524,8FC1D4,DE3D61\n3525,8FC205,1E3B40\n3526,8FC246,1E3F81\n3527,8FC277,1E30A0\n3528,8FC2C0,DE32C1\n3529,8FC2F1,1E3FA0\n3530,8FC33A,1E4380\n3531,8FC4F5,1E3C21\n3532,8FC538,1E3B80\n3533,8FC569,1E3F60\n3534,8FC5B2,DE30C0\n3535,8FC819,1E4F01\n3536,8FD942,1802BC0\n3537,8FDBB1,1803220\n3538,8FEC78,1E4640\n3539,8FED5F,1E4BA0\n3540,8FEE8A,1E3801\n3541,8FEF15,1E3E20\n3542,8FEFF4,1E3921\n3543,8FF111,1E34E0\n3544,8FF1A2,1E33C0\n3545,8FF1EB,1E36E1\n3546,8FF248,1E3701\n3547,8FF35F,1E3461\n3548,8FF3A8,1E3E20\n3549,8FFE3D,BE3381\n3550,8FFE86,BE3240\n3551,9078AF,1FE39A0\n3552,9078F8,1FE3E01\n3553,90FF3B,BE33A0\n3554,9100B8,BE3420\n3555,9100FF,BE33E1\n3556,929630,1FE3280\n3557,929677,1FE3AC0\n3558,9296C0,1FE3AC0\n3559,929707,1FE3681\n3560,929742,1FE36A0\n3561,929791,1FE5180\n3562,9297DA,1FE4001\n3563,92981F,1FE3DA1\n3564,929856,1FE3401\n3565,92988B,1FE3981\n3566,9298CA,1FE4181\n3567,9298FB,1FE36A0\n3568,92992E,DE3600\n3569,92995F,1FE4141\n3570,929992,7E3EC1\n3571,9299C3,1FE4361\n3572,9299F6,7E3A60\n3573,929A5B,1FE3000\n3574,929AC6,1FE5261\n3575,92B815,1802C20\n3576,92BC9C,1802EA0\n3577,92BD2F,1802D21\n3578,92BF6A,1802E60\n3579,92C427,5E3640\n3580,92C5A4,1E39A0\n3581,92C5D5,5E3DE1\n3582,92C608,DE3BA1\n3583,92C639,5E3520\n3584,92CA4C,1E34C1\n3585,92CCDD,1E3740\n3586,92CD70,1E34E0\n3587,92CE07,1E3DE0\n3588,92CE58,1E43A1\n3589,92CE9F,1E3AA0\n3590,92CEE8,1E3D80\n3591,92CF2F,1E4121\n3592,92CFD8,1E3AC0\n3593,92D041,1E3B40\n3594,92D088,DE3B61\n3595,92D0B9,1E4F20\n3596,92D116,1E3F00\n3597,92D147,1E3CC0\n3598,92D1C6,1E3D61\n3599,92D207,1E37A1\n3600,92D33E,1E3C21\n3601,92D3EB,1E3FC0\n3602,92D53C,1E4721\n3603,92D5F3,1E4160\n3604,92DAAE,1802B81\n3605,92E19B,1802DE1\n3606,92F8FE,1E3C41\n3607,92FAD5,1E3BE0\n3608,92FC68,1E34C1\n3609,92FC99,1E3161\n3610,930BD2,BE3480\n3611,930CC7,5E3380\n3612,9414CC,BE3420\n3613,94153D,BE3A81\n3614,941586,BE3681\n3615,94162B,BE33E1\n3616,941796,BE3240\n3617,95A5A1,1FE3761\n3618,95A5FE,1FE35A0\n3619,95A62F,1FE3541\n3620,95A66C,1FE41E1\n3621,95A69D,7E3AC0\n3622,95A6D0,1FE4961\n3623,95A701,DE3280\n3624,95A734,1FE3CA0\n3625,95A76B,1FE45A1\n3626,95A79E,1FE3B40\n3627,95A7CF,DE3941\n3628,95A802,1FE5300\n3629,95C6AF,1802DC0\n3630,95C6FA,1803480\n3631,95C89B,1802D41\n3632,95D232,5E3160\n3633,95D597,18032E0\n3634,95D740,1E3461\n3635,95D771,1E35C0\n3636,95D922,1E3641\n3637,95D953,1E3B01\n3638,95D9A8,1E35C0\n3639,95D9F1,1E4061\n3640,95DA3C,1E3560\n3641,95DAE5,1E3981\n3642,95DB28,1E3780\n3643,95DB8F,1E3720\n3644,95DBD8,1E4121\n3645,95DC25,1E36C0\n3646,95DC64,1E3780\n3647,95DCAB,DE39A0\n3648,95DCDE,1E4FE0\n3649,95DD39,1E36E1\n3650,95DD6C,1E3921\n3651,95DDA9,1E3341\n3652,95DDE2,1E3820\n3653,95DE13,DE3180\n3654,95DE64,1E4281\n3655,95DE95,1E3C41\n3656,95DED8,1E4481\n3657,95DFC5,1E3AC0\n3658,95E012,1E5041\n3659,95E1C9,1E4460\n3660,95E3D2,1E3A00\n3661,95F345,1801CC1\n3662,9605D2,1E35A0\n3663,960645,1E3621\n3664,9607BC,1E4441\n3665,96087B,1E33E1\n3666,960976,1E3AC0\n3667,9609C5,1E38A1\n3668,960C24,1E3660\n3669,96182F,BE3521\n3670,969324,1FE30C0\n3671,969373,1FE3560\n3672,9693C2,1FE4361\n3673,971E91,BE3140\n3674,972004,BE30E1\n3675,97204B,BE37C1\n3676,9722A4,BE3120\n3677,9722DF,BE3060\n3678,98B0F2,1FE3880\n3679,98B13B,1FE3500\n3680,98B182,1FE3500\n3681,98B1CB,1FE3461\n3682,98B21C,1FE3A21\n3683,98B24D,1FE3B80\n3684,98B28C,1FE34A1\n3685,98B2BD,1FE3600\n3686,98B2F0,DE3600\n3687,98B321,1FE41A0\n3688,98B35E,1FE37E0\n3689,98B395,1FE34C1\n3690,98B3CC,1FE3660\n3691,98B401,1FE3420\n3692,98B434,DE37A1\n3693,98B47F,7E3761\n3694,98B4B2,1FE3F41\n3695,98B4E3,7E3AE1\n3696,98B51C,1FE46C1\n3697,98B54D,7E38E0\n3698,98B580,DE3C00\n3699,98DF4F,5E32C0\n3700,98DFFA,5E32E1\n3701,98E043,1E35C0\n3702,98E08C,1802D41\n3703,98E13B,1E3801\n3704,98E16E,1803081\n3705,98E19F,1E3401\n3706,98E1D2,1E3500\n3707,98E22D,1E3AC0\n3708,98E260,1803140\n3709,98E2F7,1E38A1\n3710,98E436,1E3480\n3711,98E475,1E3B80\n3712,98E4C2,1E33E1\n3713,98E4F3,1E3861\n3714,98E53A,DE3401\n3715,98E56B,1803161\n3716,98E59E,1E35A0\n3717,98E5CF,18028A0\n3718,98E602,1E3A41\n3719,98E63B,1E3820\n3720,98E66E,18030E1\n3721,98E69F,DE3EE0\n3722,98E6D2,1E3440\n3723,98E703,1E3660\n3724,98E74C,1E34E0\n3725,98E77D,1E3EC1\n3726,98E7BA,1E4061\n3727,98E7EB,DE4260\n3728,98E828,1E3AA0\n3729,98E905,1E2E00\n3730,98EA36,1802BE1\n3731,98EA67,1E36A0\n3732,98EAD2,1E36A0\n3733,98EB85,1E4400\n3734,9917B0,1E3DC1\n3735,991A8D,1E36E1\n3736,991B00,1E33A0\n3737,991B31,1E3900\n3738,991B7C,DE36A0\n3739,991C0D,1E3600\n3740,991CC8,1E3360\n3741,99261B,BE3420\n3742,99268E,BE32C1\n3743,9926C3,BE36A0\n3744,992706,BE3420\n3745,992743,DE32A1\n3746,99A106,1FE4020\n3747,99A137,1FE2320\n3748,99A186,1FE3C60\n3749,99A1CD,1FE3541\n3750,99A21C,1FE35A0\n3751,9A230F,BE3300\n3752,9A25A2,BE3321\n3753,9A285D,BE3801\n3754,9BBF76,1FE3B20\n3755,9BBFBD,1FE4AA1\n3756,9BC006,1FE3F00\n3757,9BC045,1FE3401\n3758,9BC07C,1FE35C0\n3759,9BC0AF,1FE3761\n3760,9BC0EC,1FE3F81\n3761,9BC11F,1FE2FC1\n3762,9BC15A,1FE4320\n3763,9BC18B,1FE37A1\n3764,9BC1BE,DE3740\n3765,9BC1EF,1FE38C1\n3766,9BC228,1FE4061\n3767,9BC275,7E3720\n3768,9BC2A8,1FE4441\n3769,9BC2D9,7E34E0\n3770,9BC312,1FE4860\n3771,9BC343,DE4F01\n3772,9BC376,7E3981\n3773,9BE44D,1802D81\n3774,9BE612,1802D21\n3775,9BEA65,1802FE0\n3776,9BEC5A,5E3181\n3777,9BECE5,1E38A1\n3778,9BEE42,5E3020\n3779,9BEE89,5E3501\n3780,9BEEBC,5E34A0\n3781,9BF085,1E35C0\n3782,9BF0FC,1E3401\n3783,9BF17F,1E3B40\n3784,9BF1C6,1E4001\n3785,9BF273,1E39E1\n3786,9BF2AA,1E3300\n3787,9BF2DB,DE3CA0\n3788,9BF30E,1E3861\n3789,9BF355,1E3440\n3790,9BF38C,1E32A1\n3791,9BF3D3,1E3660\n3792,9BF416,1E4221\n3793,9BF447,1E3DE0\n3794,9BF480,1E36C0\n3795,9BF4C7,1E4020\n3796,9BF4FA,1E3780\n3797,9BF571,DE32E0\n3798,9BF5A4,1E3820\n3799,9BF5E5,1E3600\n3800,9BF642,1E3B01\n3801,9BF68B,1E3F21\n3802,9BF7AA,1E3861\n3803,9BF823,1E3820\n3804,9C03B4,1803300\n3805,9C2725,1E3C41\n3806,9C27C2,1E3861\n3807,9C28DB,1E4020\n3808,9C290E,1E3581\n3809,9C293F,DE3AE1\n3810,9C2972,1E36C0\n3811,9C29C1,1E3521\n3812,9C29F4,1E3820\n3813,9C2A3D,DE3560\n3814,9C2A70,1E3720\n3815,9C2AA1,1E3BC1\n3816,9C2CFC,1E3300\n3817,9C3245,BE3280\n3818,9C328E,BE3701\n3819,9C334D,BE3220\n3820,9CADC6,1FE2C61\n3821,9CAE21,1FE2821\n3822,9CAE72,1FE3B80\n3823,9CAEBB,1FE3BA1\n3824,9D3B16,BE33E1\n3825,9D3B73,BE2980\n3826,9D3BBC,BE3461\n3827,9D3BF3,BE2F20\n3828,9D3C30,BE3861\n3829,9D3C69,BE3461\n3830,9D3C9C,DE3761\n3831,9D3CD7,BE3321\n3832,9D3D20,BE3280\n3833,9D3D91,BE31A1\n3834,9D3DD4,DE39A0\n3835,9D3F33,BE3381\n3836,9D3F72,BE3261\n3837,9D405B,BE31A1\n3838,9D41CC,BE31C1\n3839,9ECD57,1FE3981\n3840,9ECDC0,1FE3621\n3841,9ECE0F,DE34C1\n3842,9ECE42,1FE3681\n3843,9ECE8D,1FE5081\n3844,9ECEDC,1FE5401\n3845,9ECF21,7E37A1\n3846,9ECF54,1FE5161\n3847,9ECF85,DE36E1\n3848,9ECFB8,7E37E0\n3849,9EF193,1803140\n3850,9EF78E,1802C01\n3851,9EF867,1802DE1\n3852,9EF96E,18030A0\n3853,9EFD7F,5E3460\n3854,9F0038,1E3880\n3855,9F0143,1E3820\n3856,9F0284,1E3880\n3857,9F0359,1E3541\n3858,9F039A,1E4721\n3859,9F0405,1E3440\n3860,9F0446,1E36C0\n3861,9F0477,DE39A0\n3862,9F04AA,1E37E0\n3863,9F04DB,1E3461\n3864,9F0580,1E3900\n3865,9F05C7,1E4080\n3866,9F060E,1E39A0\n3867,9F064F,1E3F81\n3868,9F0682,1E3E80\n3869,9F06C9,DE38A1\n3870,9F06FE,1E3A41\n3871,9F072F,1E3AE1\n3872,9F0768,1E3641\n3873,9F07A9,1E4160\n3874,9F07F2,1E4160\n3875,9F0823,1E4061\n3876,9F087A,1E3AC0\n3877,9F08AB,1E3A60\n3878,9F08EE,1E3C81\n3879,9F0993,1E3C21\n3880,9F09D4,1E3840\n3881,9F0A05,1E3D61\n3882,9F0A40,1E3641\n3883,9F0AA9,1E3C60\n3884,9F0AE6,1E3A81\n3885,9F0B17,DE3440\n3886,9F0B52,1E3941\n3887,9F0BB9,1E3840\n3888,9F0C02,DE36E1\n3889,9F0C33,1E34C1\n3890,9F0EDE,1E5CA0\n3891,9F1517,1802F80\n3892,9F16F0,1803161\n3893,9F2AF9,1E3FC0\n3894,9F2D1C,1E33C0\n3895,9F2DB9,1E35C0\n3896,9F2E04,1E3C21\n3897,9F2E45,1E3CE1\n3898,9F2E86,DE3461\n3899,9F2EB7,1E3681\n3900,9F2F72,1E3500\n3901,9F311D,1E35A0\n3902,9F3312,1E39C0\n3903,9F3F9B,BE3A00\n3904,9F4046,BE31C1\n3905,9F41F9,5E33A1\n3906,9FBB6A,1FE3B40\n3907,9FBC0B,1FE3801\n3908,9FBC56,1FE3300\n3909,A04375,BE31E0\n3910,A0464C,BE3381\n3911,A048DD,BE36E1\n3912,A1DA98,1FE35A0\n3913,A1DAC9,1FE3701\n3914,A1DAFC,1FE4980\n3915,A1DB43,1FE5560\n3916,A1DB82,1FE37E0\n3917,A1DBB3,1FE3381\n3918,A1DBE6,DE3621\n3919,A1DC17,1FE37C1\n3920,A1DC4A,7E3581\n3921,A1DC7B,1FE4520\n3922,A1DCAE,7E3B40\n3923,A1DCDF,1FE37E0\n3924,A1DD16,1FE3BA1\n3925,A1DD47,DE38C1\n3926,A1DDB2,1FE4D41\n3927,A2001B,1802CC1\n3928,A200AC,1803101\n3929,A20647,5E35C1\n3930,A2069A,5E3460\n3931,A206E9,1803000\n3932,A20758,5E36A1\n3933,A20D11,1E3DE0\n3934,A20ED4,1802B81\n3935,A20F3F,1E3AA0\n3936,A20F8E,1E3AC0\n3937,A20FE7,1E35C0\n3938,A2101A,1E36A0\n3939,A2104B,1E3641\n3940,A2109A,DE3BA1\n3941,A210CB,1E3EC1\n3942,A210FE,1E3581\n3943,A21145,1E4141\n3944,A21186,1E3880\n3945,A211CF,1E4FA1\n3946,A2120E,1E3600\n3947,A21241,1E3A41\n3948,A2128A,1E3900\n3949,A212C3,1E38E0\n3950,A2134E,1E46E0\n3951,A21437,1E3461\n3952,A21534,1E4B41\n3953,A2159F,1E4C40\n3954,A2175C,1E49C1\n3955,A23D2D,1E3A60\n3956,A23D60,1E3720\n3957,A23F95,1E3C81\n3958,A24034,1E3560\n3959,A2407D,1E37E0\n3960,A243D6,1E3581\n3961,A24ED9,BE3360\n3962,A35528,BE3201\n3963,A3559D,BE34E0\n3964,A355DC,BE33A0\n3965,A35623,BE34A1\n3966,A3580C,BE31C1\n3967,A35847,BE31A1\n3968,A3593A,BE3440\n3969,A4E6E7,1FE34E0\n3970,A4E734,1FE3DE0\n3971,A4E77F,1FE40E0\n3972,A4E7BC,1FE34E0\n3973,A4E805,1FE3F41\n3974,A4E838,1FE3321\n3975,A4E87F,1FE3E01\n3976,A4E8B2,1FE3CE1\n3977,A4E8F9,1FE55A0\n3978,A4E92C,1FE38E0\n3979,A4E95D,DE38A1\n3980,A4E990,1FE3EA1\n3981,A4E9C1,7E3401\n3982,A4E9F4,1FE5081\n3983,A4EA2D,1FE3FE1\n3984,A4EA60,1FE4421\n3985,A4EA91,DE3DE0\n3986,A4EAC4,7E39E1\n3987,A504B9,1802DC0\n3988,A50BEE,1802E41\n3989,A50D29,18031E0\n3990,A50D6E,1802D81\n3991,A5111B,1803101\n3992,A51786,5E31A0\n3993,A517B7,5E35A1\n3994,A51872,5E3481\n3995,A5193D,1E38A1\n3996,A51B08,1E3A00\n3997,A51B47,1E40A1\n3998,A51B7A,1E3381\n3999,A51BAB,DE3C21\n4000,A51C1C,1E3DE0\n4001,A51C63,1E3D01\n4002,A51CA6,1E3B20\n4003,A51CD7,1E3560\n4004,A51D1E,1E3960\n4005,A51D57,1E3500\n4006,A51D8A,1E39C0\n4007,A51DD1,DE3641\n4008,A51E04,1E3381\n4009,A51E35,DE35A0\n4010,A51E68,1E4640\n4011,A51EAF,1E4DA0\n4012,A51EE2,1E3681\n4013,A52011,1E4121\n4014,A52044,1E3A00\n4015,A520B7,1E3780\n4016,A53302,1803081\n4017,A5344F,18020A1\n4018,A54CF6,1E34A1\n4019,A54E0D,1E3A00\n4020,A54E40,1E3A41\n4021,A54E71,1E3660\n4022,A54EA4,1E3660\n4023,A54F39,1E3681\n4024,A54FD6,1E3681\n4025,A55007,1E37C1\n4026,A55064,1E4260\n4027,A55B13,BE3360\n4028,A55B54,BE34A1\n4029,A55B8D,BE3021\n4030,A55BCA,BE35A0\n4031,A55C01,BE30C0\n4032,A55C46,DE3DE0\n4033,A65C5F,BE3240\n4034,A65D4C,BE37A1\n4035,A6600D,BE32E0\n4036,A7F444,1FE38E0\n4037,A7F48F,1FE34E0\n4038,A7F4D8,1FE3AC0\n4039,A7F51F,1FE3BA1\n4040,A7F552,1FE3660\n4041,A7F591,DE3300\n4042,A7F5C4,1FE34C1\n4043,A7F607,1FE3300\n4044,A7F63A,1FE3521\n4045,A7F683,1FE4800\n4046,A7F6B6,1FE4860\n4047,A7F6E7,7E36E1\n4048,A7F71A,1FE4A01\n4049,A7F74B,DE4080\n4050,A7F784,1FE4BE1\n4051,A81659,18030C0\n4052,A816C6,1803041\n4053,A817C5,1803041\n4054,A819BE,1802CC1\n4055,A820C7,5E31A0\n4056,A82136,5E3B00\n4057,A822B7,1E3600\n4058,A826C4,1E37A1\n4059,A828F1,1E3CA0\n4060,A829EE,1E3420\n4061,A82A4B,1E37E0\n4062,A82A94,1E4061\n4063,A82ADD,1E33E1\n4064,A82BA6,1E34A1\n4065,A82BD7,1E3960\n4066,A82C1E,1E3560\n4067,A82CBF,1E35A0\n4068,A82CF2,1E3B40\n4069,A82D23,DE3360\n4070,A82D56,1E3660\n4071,A82D87,DE3500\n4072,A82DD6,1E40A1\n4073,A82E07,1E3660\n4074,A82E50,DE33E1\n4075,A82E81,1E3C60\n4076,A82EC2,1E3420\n4077,A82F8D,1E3FE1\n4078,A83062,1E3E40\n4079,A83093,1E3681\n4080,A830D0,1E4221\n4081,A83117,DE4421\n4082,A8314A,1E5360\n4083,A831B9,1E38A1\n4084,A85862,1E33E1\n4085,A859B7,1E3DC1\n4086,A859EA,1E3761\n4087,A85A1B,DE3541\n4088,A85A6C,1E3761\n4089,A85A9D,1E3300\n4090,A85AE6,1E3600\n4091,A85B89,1E3840\n4092,A85BBC,1E3660\n4093,A85C0D,1E39C0\n4094,A86880,BE33A0\n4095,A8692B,BE31E0\n4096,A96C5A,BE36C0\n4097,A96DAB,BE3440\n4098,A96E28,BE2260\n4099,A9703F,BE3381\n4100,AB0282,1FE37A1\n4101,AB02C1,1FE3360\n4102,AB02F4,1FE2F40\n4103,AB032F,1FE3840\n4104,AB0362,DE3EE0\n4105,AB0393,1FE3A21\n4106,AB03D2,1FE3E61\n4107,AB0403,1FE3F60\n4108,AB043E,1FE3E20\n4109,AB046F,1FE3CE1\n4110,AB04A2,7E34C1\n4111,AB04D3,1FE4DE1\n4112,AB0506,DE3560\n4113,AB0537,1FE4800\n4114,AB056A,7E3521\n4115,AB24B9,1802EC0\n4116,AB2B2C,18034E0\n4117,AB2D71,1802E00\n4118,AB2DBE,1E36C0\n4119,AB2F43,5E3501\n4120,AB2F94,1802EC0\n4121,AB318D,5E3241\n4122,AB32C2,5E3460\n4123,AB357D,1E3761\n4124,AB35CC,1E3C21\n4125,AB36B9,1E4241\n4126,AB36EC,1E3641\n4127,AB3763,1E3B80\n4128,AB37AC,1E3740\n4129,AB3881,1E35A0\n4130,AB38B4,1E35E1\n4131,AB3949,1E3801\n4132,AB398C,1E38A1\n4133,AB39C1,1E3C60\n4134,AB39FA,1E35A0\n4135,AB3A2B,1E3861\n4136,AB3A74,1E37A1\n4137,AB3AAD,DE3280\n4138,AB3B9E,1E3780\n4139,AB3BDF,1E4821\n4140,AB3C12,1E4741\n4141,AB3CB1,1E3F41\n4142,AB3CE4,1E3B40\n4143,AB3D1B,1E4241\n4144,AB3D68,DE3B01\n4145,AB3DFF,1E37C1\n4146,AB3E46,1E3641\n4147,AB3EDF,1E54E0\n4148,AB6586,1E3861\n4149,AB67A9,1E3641\n4150,AB6836,1E3720\n4151,AB6911,1E3581\n4152,AB6B98,1E3240\n4153,AB77AF,BE3180\n4154,AB7850,BE2DA0\n4155,ABDC35,7E3401\n4156,AC71B2,BE3240\n4157,AC71F9,BE3541\n4158,AC7358,BE31C1\n4159,AC739F,BE3081\n4160,AC7494,BE38C1\n4161,AC7743,BE2F61\n4162,AE0F5A,1FE3560\n4163,AE0FA9,1FE4640\n4164,AE0FF0,1FE3500\n4165,AE1037,1FE3FA0\n4166,AE1080,1FE40C1\n4167,AE10B3,1FE4601\n4168,AE10FC,1FE44C0\n4169,AE112D,1FE3780\n4170,AE1168,1FE32C1\n4171,AE119F,1FE3D20\n4172,AE11EC,DE3600\n4173,AE121D,1FE46E0\n4174,AE1258,1FE4320\n4175,AE12A7,7E34C1\n4176,AE2CDA,1802E81\n4177,AE30AD,1802D41\n4178,AE3158,1802D81\n4179,AE3369,1802CE0\n4180,AE3456,1802DE1\n4181,AE3CC9,5E37C0\n4182,AE3CFE,5E2021\n4183,AE3D77,5E31A0\n4184,AE3DBE,DE35E1\n4185,AE46F9,1E3C00\n4186,AE48C2,1E3840\n4187,AE4901,1E3660\n4188,AE4950,1E3C41\n4189,AE4A7B,1E4961\n4190,AE4AAE,1E3A60\n4191,AE4AF7,DE3801\n4192,AE4B2A,1E37A1\n4193,AE4B7D,1E38C1\n4194,AE4BBE,1E38C1\n4195,AE4BFD,1E3C00\n4196,AE4C32,1E3261\n4197,AE4C63,DE3941\n4198,AE4C96,1E3461\n4199,AE4CD1,1E3681\n4200,AE4D04,1E3440\n4201,AE4D3F,1E3A21\n4202,AE4D88,DE46C1\n4203,AE4DB9,1E4160\n4204,AE4DEC,1E35A0\n4205,AE4E29,1E3FA0\n4206,AE4E72,1E33C0\n4207,AE4EDF,1E3AA0\n4208,AE4F8A,1E35A0\n4209,AE4FBB,1E4100\n4210,AE4FF2,1E3480\n4211,AE503D,DE3DC1\n4212,AE5070,1E3981\n4213,AE50DB,1E3660\n4214,AE514C,1E3FA0\n4215,AE5193,DE33C0\n4216,AE51C6,1E3880\n4217,AE51F7,1E30E1\n4218,AE6DC6,1E3500\n4219,AE6E0F,1E43A1\n4220,AE6E48,1E3FC0\n4221,AE6F4F,1E35E1\n4222,AE6F82,1E3480\n4223,AE6FC1,1E3461\n4224,AE6FFC,DE3921\n4225,AE702D,1E3960\n4226,AE7116,1E3CC0\n4227,AE715D,1E3EE0\n4228,AE71A6,1E36A0\n4229,AE7215,1E35A0\n4230,AE7340,1E3C21\n4231,AE8577,BE3161\n4232,AE85C0,BE3780\n4233,AE8665,BE3A21\n4234,AF85B0,BE37C1\n4235,AF85F7,BE33A0\n4236,AF879E,BE33C0\n4237,AF87E5,BE3261\n4238,AF88D6,BE32C1\n4239,AF8A75,BE3401\n4240,B11C8C,1FE38C1\n4241,B11CD3,1FE4680\n4242,B11D1E,1FE3641\n4243,B11D69,1FE3B20\n4244,B11D9C,1FE37E0\n4245,B11DE3,1FE3B20\n4246,B11E16,1FE3981\n4247,B11E51,1FE3701\n4248,B11E84,1FE3641\n4249,B11EB5,DE4100\n4250,B11EE8,1FE3E20\n4251,B11F23,1FE39C0\n4252,B11F56,1FE4AC1\n4253,B11F91,1FE4580\n4254,B11FC4,7E34E0\n4255,B11FF5,DE39A0\n4256,B12028,1FE4D41\n4257,B12059,7E3480\n4258,B1208E,1FE3DA1\n4259,B13CCD,1802E41\n4260,B140DC,1802CC1\n4261,B149A5,5E3260\n4262,B14CBC,1E3A00\n4263,B14D09,1E3A81\n4264,B14F9C,1E3641\n4265,B1501B,1E35C0\n4266,B1504E,1E3321\n4267,B150C7,1E3C00\n4268,B15174,1E3C21\n4269,B151E3,1E3D40\n4270,B15216,1E3840\n4271,B1524D,1E3701\n4272,B1528E,1E3880\n4273,B152D7,1E3B20\n4274,B1531E,1E3681\n4275,B1534F,1E4580\n4276,B1538A,1E37C1\n4277,B153BB,1E3D01\n4278,B15404,1E3480\n4279,B15437,1E3EA1\n4280,B1546A,1E4061\n4281,B1549B,DE4361\n4282,B154CE,1E3FC0\n4283,B15565,1E39A0\n4284,B15598,1E35C0\n4285,B155D7,DE3581\n4286,B1560A,1E4BA0\n4287,B15659,1E46A1\n4288,B1568C,1E4320\n4289,B156C5,1E44E1\n4290,B15770,1E3880\n4291,B1692D,1802D60\n4292,B1808C,1E3A81\n4293,B18195,1E3FE1\n4294,B181DE,1E38A1\n4295,B182C7,1E3740\n4296,B183A0,1E37E0\n4297,B1840B,1E3A21\n4298,B1929C,BE3480\n4299,B20BED,1FE3A60\n4300,B20C36,1FE3900\n4301,B20C7F,1FE37C1\n4302,B20CD0,1FE3641\n4303,B29939,BE32C1\n4304,B2997A,BE34E0\n4305,B299C1,BE3240\n4306,B29BEA,BE32E0\n4307,B42A9D,1FE3581\n4308,B42AD0,1FE2F80\n4309,B42B09,1FE3581\n4310,B42B52,1FE45A1\n4311,B42B83,1FE3761\n4312,B42BCA,DE3500\n4313,B42BFB,1FE5480\n4314,B42C2E,DE3401\n4315,B42C5F,1FE3621\n4316,B42C92,7E36E1\n4317,B42CC3,1FE42E1\n4318,B42D44,7E3161\n4319,B446E9,1802CA1\n4320,B448F6,1802CA1\n4321,B44AAF,1801CE0\n4322,B44E66,1802E41\n4323,B455D7,5E32A0\n4324,B45794,5E3520\n4325,B45863,5E3680\n4326,B458E2,1E34E0\n4327,B45C45,1E3461\n4328,B45FD2,1E3900\n4329,B46015,1E3600\n4330,B461B6,1E41A0\n4331,B46201,1E4121\n4332,B46242,1E3801\n4333,B46291,1E3720\n4334,B462D2,1E33E1\n4335,B4630D,1E4281\n4336,B46356,1E3820\n4337,B463C1,1E3AC0\n4338,B463F4,1E3981\n4339,B46449,1E4061\n4340,B4647C,1E32C1\n4341,B464B1,1E3B01\n4342,B47F34,1802E21\n4343,B48D73,1E3240\n4344,B48DE0,1E3B61\n4345,B48E5F,1E39A0\n4346,B48F1C,1E3B61\n4347,B48F9B,1E3321\n4348,B48FCE,1E3BE0\n4349,B49017,1E37E0\n4350,B4904A,1E3600\n4351,B4907B,DE3240\n4352,B490AE,1E36E1\n4353,B49109,1E3681\n4354,B4913C,1E3341\n4355,B4917F,1E3720\n4356,B491C6,DE3321\n4357,B4A04B,BE3840\n4358,B59ED8,BE26C1\n4359,B59F15,BE3401\n4360,B59F5E,BE32E0\n4361,B59FDB,BE34C1\n4362,B5A0FE,BE31A1\n4363,B5A179,BE2800\n4364,B736F2,1FE34C1\n4365,B73739,1FE3B80\n4366,B73782,1FE3820\n4367,B737CB,1FE4221\n4368,B73812,1FE3D40\n4369,B73851,1FE36C0\n4370,B73890,1FE3500\n4371,B738CF,1FE3681\n4372,B73902,1FE3660\n4373,B7393B,1FE3D80\n4374,B7396E,1FE3740\n4375,B7399F,7E37C1\n4376,B739D2,1FE5360\n4377,B73A03,DE3DA1\n4378,B73A36,1FE3DA1\n4379,B73A67,7E35E1\n4380,B73A9A,1FE38C1\n4381,B73AE5,DE3101\n4382,B752B2,1802D81\n4383,B75409,1802F20\n4384,B754C8,1802CA1\n4385,B7680B,5E39A1\n4386,B76852,5E3441\n4387,B7689B,5E3400\n4388,B768E6,5E32A0\n4389,B76935,5E37A0\n4390,B76A16,5E3760\n4391,B76BD5,1E3641\n4392,B76D9C,1E3C60\n4393,B76DE1,1E4241\n4394,B7710A,1E3600\n4395,B77151,1E3BC1\n4396,B7719A,1E4400\n4397,B771EB,1E3740\n4398,B77220,1E3AC0\n4399,B77251,1E4741\n4400,B77284,DE3140\n4401,B772B5,1E3900\n4402,B772EC,1E34C1\n4403,B7732D,1E3720\n4404,B77376,1E3C81\n4405,B773BF,1E4340\n4406,B773FE,1E3820\n4407,B77441,1E3B20\n4408,B77474,1E3A00\n4409,B774A5,1E3B61\n4410,B774EE,1E38C1\n4411,B7751F,DE3381\n4412,B77552,1E3FA0\n4413,B77583,1E4D00\n4414,B775CC,1E38A1\n4415,B77607,1E3900\n4416,B77652,DE3AC0\n4417,B77683,1E3880\n4418,B7780E,1E3E61\n4419,B778F9,1E3EE0\n4420,B789AC,1802D81\n4421,B79745,1E4020\n4422,B797C8,1E3A81\n4423,B79811,1E39E1\n4424,B7984C,1E3041\n4425,B798F3,1E3921\n4426,B7998E,1E38C1\n4427,B79AA9,1E3381\n4428,B79ADC,1E3581\n4429,B79B0D,1E3DC1\n4430,B79B56,DE33A0\n4431,B79B87,1E3C21\n4432,B79BFE,1E3480\n4433,B7ACB3,BE3240\n4434,B7ACF0,BE3801\n4435,B7AD35,BE35E1\n4436,B7AD6E,BE30C0\n4437,B7ADA9,BE38C1\n4438,B7ADEC,DE3720\n4439,B826FD,1FE3401\n4440,B82748,1FE32E0\n4441,B82797,1FE4020\n4442,B8A700,BE3360\n4443,B8A83D,BE3440\n4444,B8A8EA,BE3201\n4445,B8AA01,BE3641\n4446,B8AF0A,BE3440\n4447,B8AF51,1FE3641\n4448,BA4482,1FE38C1\n4449,BA44CB,1FE3600\n4450,BA4514,1FE3FC0\n4451,BA455B,1FE3EE0\n4452,BA45A2,1FE3AA0\n4453,BA45DB,1FE31A1\n4454,BA461E,1FE3420\n4455,BA464F,1FE3840\n4456,BA4696,1FE5101\n4457,BA46CB,1FE3801\n4458,BA4702,1FE32C1\n4459,BA4733,DE3861\n4460,BA4766,1FE34C1\n4461,BA4797,7E3621\n4462,BA47CA,1FE4460\n4463,BA4805,1FE3C41\n4464,BA4838,7E3BE0\n4465,BA4869,1FE4F61\n4466,BA489C,DE3720\n4467,BA6D2D,1802BC0\n4468,BA6F70,1802FC1\n4469,BA70A9,1802C01\n4470,BA7206,5E31C0\n4471,BA7293,1E3761\n4472,BA72C6,5E3441\n4473,BA742F,5E3361\n4474,BA747E,1E3AC0\n4475,BA74AF,1E3A00\n4476,BA74E2,1E3CA0\n4477,BA7529,1E39A0\n4478,BA756C,DE33C0\n4479,BA759D,1E3C00\n4480,BA762E,1E3C21\n4481,BA767D,1E3D80\n4482,BA76B0,1E3900\n4483,BA772D,1E3761\n4484,BA7760,1E3F60\n4485,BA77A9,1E3A81\n4486,BA77DC,1E4620\n4487,BA7819,DE3521\n4488,BA784C,1E3641\n4489,BA78CD,1E36C0\n4490,BA7950,1E3641\n4491,BA7997,1E3AE1\n4492,BA79CA,1E4160\n4493,BA7AD1,1E4640\n4494,BA7B3A,1E4BA0\n4495,BA7B77,1E3A60\n4496,BA7BC0,1E4F61\n4497,BA7BF1,1E4561\n4498,BA7C26,1E3621\n4499,BA7CF7,1E4520\n4500,BAACF2,1E3EC1\n4501,BAAD73,1E4160\n4502,BAAE90,1E3581\n4503,BAAEFF,1E4020\n4504,BAAF48,1E3761\n4505,BAB0FB,1E3641\n4506,BABB96,BE3440\n4507,BABBDD,BE3720\n4508,BABC16,BE32E0\n4509,BABC4B,BE31A1\n4510,BABC8E,BE3BC1\n4511,BABCBF,5E3501\n4512,BABCF2,DE4320\n4513,BB3407,1FE3600\n4514,BB3452,1FE3E80\n4515,BB3493,1FE35A0\n4516,BB34DE,1FE3D20\n4517,BB3539,1FE3161\n4518,BBB5C4,BE36E1\n4519,BBB8A7,BE3321\n4520,BBB9DC,BE33C0\n4521,BBBB17,BE33C0\n4522,BBC0A6,BE2F80\n4523,BD5299,1FE3261\n4524,BD52E2,1FE3EE0\n4525,BD531F,1FE3C41\n4526,BD5356,1FE3440\n4527,BD538B,1FE3560\n4528,BD53BE,DE37E0\n4529,BD53EF,1FE3621\n4530,BD542C,1FE36C0\n4531,BD545D,7E35C0\n4532,BD5490,1FE35C0\n4533,BD54C1,DE3480\n4534,BD54F4,7E31E0\n4535,BD5525,7E3840\n4536,BD7868,1802D81\n4537,BD7C0F,1802C40\n4538,BD7F14,1802F01\n4539,BD8027,5E3520\n4540,BD8090,5E3221\n4541,BD80CD,5E3421\n4542,BD811C,1E37C1\n4543,BD814D,5E3001\n4544,BD8436,1E3F00\n4545,BD84A9,1E36E1\n4546,BD8512,18025E0\n4547,BD856F,1E36E1\n4548,BD85B8,1E3D20\n4549,BD85E9,1E3740\n4550,BD8646,1E3AA0\n4551,BD8691,1E3941\n4552,BD86EE,1E43E0\n4553,BD871F,1E38C1\n4554,BD875A,1E3DA1\n4555,BD879B,1E3DA1\n4556,BD87CE,1E38A1\n4557,BD87FF,1E47E1\n4558,BD8848,DE4241\n4559,BD8879,1E4E41\n4560,BD88B8,1E3D40\n4561,BD897D,1E38A1\n4562,BD89E6,1E3921\n4563,BD8A51,1E4040\n4564,BD8B5A,1E4020\n4565,BD8CE9,1E4AA1\n4566,BD8D54,1E4920\n4567,BD8D85,1802E21\n4568,BDB8D0,1E3C21\n4569,BDB941,1E37A1\n4570,BDB9AC,1E3A81\n4571,BDBA09,1E38C1\n4572,BDBA76,1E3C21\n4573,BDBBA9,1E3AC0\n4574,BDBBDC,1E3880\n4575,BDC7EB,BE3180\n4576,BDC920,BE3321\n4577,BE4165,1FE3AC0\n4578,BE41B0,1FE3F60\n4579,BE41F7,1FE39A0\n4580,BED184,BE3161\n4581,BED26B,BE3180\n4582,BED3A8,BE3220\n4583,C05F91,1FE3641\n4584,C05FE0,1FE4EC0\n4585,C06015,1FE36E1\n4586,C06060,1FE4241\n4587,C06091,1FE3660\n4588,C060D2,1FE33E1\n4589,C0610B,1FE3560\n4590,C0613E,DE36C0\n4591,C0617B,1FE3401\n4592,C061AE,7E3621\n4593,C061DF,1FE3560\n4594,C06218,1FE31E0\n4595,C06249,1FE3C21\n4596,C0627C,DE3480\n4597,C062AD,1FE4980\n4598,C062E0,7E33E1\n4599,C085CF,1802DE1\n4600,C08656,1802D60\n4601,C087B7,1802E21\n4602,C08974,1802EA0\n4603,C08B3D,1803360\n4604,C08E56,5E3320\n4605,C08EE5,1803180\n4606,C08F32,1E3840\n4607,C08F63,5E4161\n4608,C08F96,DE3101\n4609,C090CF,1E3541\n4610,C09276,1E38A1\n4611,C0933B,1E3801\n4612,C09370,1E3641\n4613,C093A1,DE3581\n4614,C093D4,1E3641\n4615,C0942D,1E3840\n4616,C0947C,1E3DC1\n4617,C094BD,DE3161\n4618,C094F0,1E3C60\n4619,C09527,1E3C21\n4620,C0955A,1E3681\n4621,C095B5,1E3C00\n4622,C09624,1E3C00\n4623,C09661,1E3740\n4624,C09696,1E33A0\n4625,C096D3,1E3780\n4626,C09732,1E39C0\n4627,C0979F,1E3420\n4628,C097E8,1E4B21\n4629,C09819,1E39A0\n4630,C0988E,1E3E01\n4631,C09B5B,1E50A0\n4632,C0A456,1802BA0\n4633,C0C793,1E31A1\n4634,C0C7DC,1E3521\n4635,C0C823,1E3660\n4636,C0C86C,1E3560\n4637,C0C8B3,1E38A1\n4638,C0D6CE,BE33A0\n4639,C0D7BB,5E2541\n4640,C14E52,1FE3701\n4641,C14EAD,1FE3D20\n4642,C14EF6,1FE3840\n4643,C14F3D,1FE3401\n4644,C14F8C,1FE3641\n4645,C14FD3,1FE3461\n4646,C1DD42,BE3261\n4647,C1DE9B,BE3401\n4648,C1DFDE,BE33E1\n4649,C36CB5,1FE3280\n4650,C36CFC,1FE4320\n4651,C36D45,1FE3921\n4652,C36D8E,1FE4281\n4653,C36DD5,1FE3FE1\n4654,C36E14,1FE35A0\n4655,C36E5B,1FE4A20\n4656,C36E9E,1FE3621\n4657,C36ECF,1FE3660\n4658,C36F0C,1FE3600\n4659,C36F3F,1FE3740\n4660,C36F76,1FE4001\n4661,C36FAD,1FE48C0\n4662,C37004,7E3600\n4663,C37035,1FE3041\n4664,C3706C,7E3681\n4665,C3709D,1FE5360\n4666,C38D80,1802FC1\n4667,C38F01,1802E60\n4668,C390CC,1803021\n4669,C399F3,5E3221\n4670,C39BA4,5E35C1\n4671,C3A0AF,1E3A21\n4672,C3A100,1E3D40\n4673,C3A285,1E3161\n4674,C3A37A,1E3560\n4675,C3A3C1,1E33E1\n4676,C3A46E,1E3E01\n4677,C3A4C9,1E3761\n4678,C3A512,1E3DC1\n4679,C3A557,1E3E40\n4680,C3A5A8,1E4040\n4681,C3A60F,1E3521\n4682,C3A642,1E3761\n4683,C3A673,1E3641\n4684,C3A6BA,1E3880\n4685,C3A6F9,1E3681\n4686,C3A73A,1E3AE1\n4687,C3A76D,1E3A81\n4688,C3A7AE,DE3EC1\n4689,C3A7DF,1E36E1\n4690,C3A812,1E3AE1\n4691,C3A859,1E3AA0\n4692,C3A89A,1E3B20\n4693,C3A925,1E4540\n4694,C3A966,1E43E0\n4695,C3A9C3,1E3780\n4696,C3AA0C,1E3261\n4697,C3AA3D,1E34A1\n4698,C3AB2C,1E38A1\n4699,C3CCB9,1E54C1\n4700,C3CE7E,1E4200\n4701,C3CEFF,1E35A0\n4702,C3CF48,1E3B40\n4703,C3CF97,1E3780\n4704,C3D03A,1E3921\n4705,C3D06B,1E3761\n4706,C3D0B4,DE3420\n4707,C3D0E5,1E38E0\n4708,C3D120,1E3720\n4709,C3D225,1E3B01\n4710,C3E1F0,BE31E0\n4711,C3E317,BE3840\n4712,C447D4,7E2E00\n4713,C45C07,1FE3641\n4714,C45C3A,1FE35C0\n4715,C45C6B,1FE3780\n4716,C45C9E,1FE3E01\n4717,C45CED,1FE37E0\n4718,C4E2E6,BE32E0\n4719,C4E445,BE3621\n4720,C4E5D0,BE21A0\n4721,C4E701,BE3161\n4722,C4E73A,BE36A0\n4723,C4E781,BE37A1\n4724,C4E830,BE3DA1\n4725,C4EAE3,BE34A1\n4726,C67AA4,1FE35A0\n4727,C67AE9,1FE3F41\n4728,C67B32,1FE3A00\n4729,C67B6D,1FE3761\n4730,C67BAA,1FE32C1\n4731,C67BF5,1FE3EE0\n4732,C67C28,1FE3641\n4733,C67C63,1FE3480\n4734,C67C98,1FE33E1\n4735,C67CC9,7E4001\n4736,C67CFC,1FE3E20\n4737,C67D35,1FE3EE0\n4738,C67D68,DE3861\n4739,C67D99,1FE3401\n4740,C67DCC,7E3C41\n4741,C67DFD,1FE4A20\n4742,C67E36,1FE4100\n4743,C67E69,1FE4D60\n4744,C67EA0,1FE3F41\n4745,C67ED1,DE3FC0\n4746,C69C86,1802EC0\n4747,C69CD1,1802E21\n4748,C69D1E,18037E0\n4749,C69E49,1803021\n4750,C69E96,1202DE1\n4751,C69EC7,1E3BE0\n4752,C6A586,1E3641\n4753,C6A7CD,5E3540\n4754,C6A918,5E3340\n4755,C6A949,1E36A0\n4756,C6A97C,5E3460\n4757,C6A9AD,1E3C81\n4758,C6AA68,1E32E0\n4759,C6AAAF,1E33A0\n4760,C6AAE8,1E3761\n4761,C6AB19,1E3621\n4762,C6AB9A,1E38C1\n4763,C6ABE3,1E3E01\n4764,C6AC44,1E3E61\n4765,C6ACB7,1E38A1\n4766,C6ACF6,1E3F41\n4767,C6AD3F,1E4520\n4768,C6B090,1E43C1\n4769,C6B0FD,1E41E1\n4770,C6CA42,18030C0\n4771,C6CC07,1802D21\n4772,C6CF6A,1802CC1\n4773,C6E59D,1E40E0\n4774,C6E768,1E3560\n4775,C6E7A3,1E3621\n4776,C6E7F2,1E3981\n4777,C6EEEF,BE37A1\n4778,C6F034,BE3401\n4779,C769A5,1FE32A1\n4780,C7F6EA,BE3440\n4781,C7F731,BE3B01\n4782,C7F780,BE3480\n4783,C7F82D,BE3480\n4784,C7FADE,BE31A1\n4785,C987FD,1FE3321\n4786,C98846,1FE4441\n4787,C98885,DE3621\n4788,C988B8,1FE39E1\n4789,C98901,1FE32A1\n4790,C98938,1FE3780\n4791,C98971,1FE31E0\n4792,C989B2,DE32C1\n4793,C989E3,1FE3201\n4794,C98A20,1FE3B80\n4795,C98A51,1FE3E20\n4796,C98A8A,1FE3921\n4797,C98AD7,7E3440\n4798,C98B0A,1FE3B20\n4799,C98B3F,1FE3960\n4800,C98B74,1FE3E80\n4801,C98BDB,1FE3C60\n4802,C98D44,1E3621\n4803,C9A453,1803201\n4804,C9A6E6,1802F80\n4805,C9B59B,5E2F60\n4806,C9B65C,5E35A1\n4807,C9B75D,1E39E1\n4808,C9B794,5E3340\n4809,C9B821,5E3580\n4810,C9BA14,1E34E0\n4811,C9BA5B,1E3FA0\n4812,C9BB04,1E39A0\n4813,C9BC0F,1E36E1\n4814,C9BC42,1E34A1\n4815,C9BCA5,1E33E1\n4816,C9BCE8,1E36E1\n4817,C9BDBF,1E3C00\n4818,C9BE5C,1E3AC0\n4819,C9BEA7,1E3DC1\n4820,C9BF12,1E4781\n4821,C9BF59,1E3F41\n4822,C9BFA2,1E3EC1\n4823,C9BFEB,1E38C1\n4824,C9C0A4,1E3081\n4825,C9C0D7,1E4361\n4826,C9C184,1E37A1\n4827,C9C203,1E3780\n4828,C9C236,1E4760\n4829,C9C27F,DE33C0\n4830,C9C3CA,1E4821\n4831,C9DC43,1802F80\n4832,C9ECAC,1E3B20\n4833,C9EE0B,1E36A0\n4834,C9EE76,1E34E0\n4835,C9EF25,1E3701\n4836,C9EF74,1E3701\n4837,C9EFBB,1E3C00\n4838,C9EFEE,1E3641\n4839,C9F09D,1E3DC1\n4840,C9F0EC,1E3A21\n4841,C9F1D7,1E35C0\n4842,C9FD14,BE32E0\n4843,C9FE31,BE32A1\n4844,C9FF38,5E33C1\n4845,CB08A5,BE3220\n4846,CB08EE,BE3480\n4847,CB09E1,BE3581\n4848,CB0F2C,BE3381\n4849,CC95C1,1FE3500\n4850,CC960A,1FE3E01\n4851,CC9653,1FE5220\n4852,CC969C,1FE3E20\n4853,CC96E3,1FE4421\n4854,CC9716,1FE3541\n4855,CC975F,DE3500\n4856,CC9792,1FE5021\n4857,CC97CB,1FE3C41\n4858,CC97FE,1FE36C0\n4859,CC982F,7E37E0\n4860,CC9862,1FE43E0\n4861,CC9893,7E36C0\n4862,CC98C6,1FE53C0\n4863,CC98F7,DE3720\n4864,CC992A,1FE49C1\n4865,CCBB03,1802F61\n4866,CCBF6E,1803220\n4867,CCC017,1802E41\n4868,CCC1EA,1802CE0\n4869,CCC4F5,5E3520\n4870,CCCA5C,1E3E40\n4871,CCCB47,1E3740\n4872,CCCB98,1E3EA1\n4873,CCCBDF,1E3420\n4874,CCCC22,1E3F81\n4875,CCCC63,DE3480\n4876,CCCDDA,1E4920\n4877,CCCE23,1E3C41\n4878,CCCE92,1E36A0\n4879,CCCED3,1E3DE0\n4880,CCCF14,DE3280\n4881,CCCF45,1E3861\n4882,CCCF86,1E3621\n4883,CCCFCD,1E3500\n4884,CCD016,1E3820\n4885,CCD091,1E3541\n4886,CCD0D8,1E5081\n4887,CCD109,1802E41\n4888,CCD13C,1E4061\n4889,CCD183,DE36A0\n4890,CCD1B6,1E4400\n4891,CCD227,1E3240\n4892,CCD25A,1E3CA0\n4893,CCD29D,1E3B61\n4894,CCD2E0,DE3AE1\n4895,CCD311,1E3BC1\n4896,CCD4D4,1E3701\n4897,CCD5D5,1E3CC0\n4898,CCDD4A,1802D00\n4899,CCE051,1802EE1\n4900,CCE5BE,1802D00\n4901,CCF5D9,1E34C1\n4902,CCF664,1E3740\n4903,CCF76B,1E3DA1\n4904,CCF7B4,1E36C0\n4905,CCF7FB,1E3820\n4906,CCF82E,1E39E1\n4907,CCF90F,1E3900\n4908,CCF942,1E3740\n4909,CCF973,DE3E80\n4910,CD0958,BE39C0\n4911,CD0A9D,BE3341\n4912,CD0B6E,BE3201\n4913,CD8473,1FE3DA1\n4914,CD84BC,1FE35A0\n4915,CD850B,1FE34C1\n4916,CD855A,1FE40E0\n4917,CE0B97,BE32C1\n4918,CE0E60,BE31C1\n4919,CE0EA7,BE3641\n4920,CE0EF0,BE32C1\n4921,CE0FAB,BE33A0\n4922,CE0FE8,BE33A0\n4923,CE102F,1FE3621\n4924,CE1062,BE3521\n4925,CE10D7,BE3861\n4926,CFA296,1FE3300\n4927,CFA2DD,1FE34A1\n4928,CFA326,1FE37E0\n4929,CFA36F,1FE3DE0\n4930,CFA3B8,1FE3560\n4931,CFA3FF,1FE41C0\n4932,CFA43E,1FE34E0\n4933,CFA487,1FE44A0\n4934,CFA4D0,1FE4361\n4935,CFA501,1FE3E80\n4936,CFA53C,1FE3420\n4937,CFA573,1FE3480\n4938,CFA5BC,1FE4C01\n4939,CFA5ED,1FE3CA0\n4940,CFA620,7E3880\n4941,CFA651,1FE3E01\n4942,CFA684,DE44E1\n4943,CFA6B5,1FE3780\n4944,CFA6E8,7E3641\n4945,CFA753,1FE4F61\n4946,CFC38E,1802E81\n4947,CFC539,1802FA1\n4948,CFCA24,1803060\n4949,CFD123,5E3821\n4950,CFD156,5E3380\n4951,CFD675,1E3761\n4952,CFD7D0,1E3621\n4953,CFD81F,1E3C41\n4954,CFD8CA,1E33E1\n4955,CFD911,1E3B20\n4956,CFD9D8,1E3A41\n4957,CFDA23,1E4460\n4958,CFDB12,1E3780\n4959,CFDB43,1E3E40\n4960,CFDB76,DE3921\n4961,CFDBA7,1E3720\n4962,CFDBDE,1E3B20\n4963,CFDC25,1E3600\n4964,CFDC6E,1E3D61\n4965,CFDCB1,1E3BE0\n4966,CFDCFA,1E3FC0\n4967,CFDD63,1E4080\n4968,CFDD98,1E4721\n4969,CFDDD3,1E3600\n4970,CFDE06,DE37E0\n4971,CFDE37,1E4141\n4972,CFDE72,1E3941\n4973,CFDEDD,1E3FE1\n4974,CFDF2C,DE3820\n4975,CFDF5D,1E4AE0\n4976,CFDFCA,1E3641\n4977,CFDFFB,1E4340\n4978,CFF0F6,1802D21\n4979,D00547,1E3960\n4980,D005E2,1E3761\n4981,D00719,1E3401\n4982,D0074C,1E3C00\n4983,D01811,BE3201\n4984,D11BD0,BE34E0\n4985,D11D35,BE32E0\n4986,D11E86,BE3521\n4987,D11FE1,BE3101\n4988,D12030,BE3401\n4989,D2B0CD,1FE3D20\n4990,D2B140,1FE3560\n4991,D2B1C5,1FE36C0\n4992,D2B234,1FE4181\n4993,D2B29F,1FE39C0\n4994,D2B2DC,7E3780\n4995,D2B30D,1FE3C21\n4996,D2B346,1FE4501\n4997,D2B3AD,1FE46A1\n4998,D2B3F6,DE3341\n4999,D2D7EB,18029A1\n") -> ("Data+Garbage"=w10:string[])  [unwired: 3 in, 1 out]
  "Array" <- w10
  n4 = Reverse String(1:w41) -> (0:w40:string)
  n5 = call "splitEveData.vi"("Clean Data Array"=w10) -> ("Energy"=→"Energy":u32[], "Channel"=w14:u32[], "Chan+Energy"=→"Chan+Energy":u32[], "Clk Ticks"=→"Clk Ticks":u32[], "Sr No"=→"Sr No":u32[])  [unwired: 3 in, 1 out]
  "Channel" <- w14
  n6 = String To Byte Array(string=w40) -> (unsigned byte array=w44:u8[])
  n7 = call "mapEventCounts.vi"("Count"=w14) -> ("Counts (map)"=w7:map{u32, u32})  [unwired: 3 in, 1 out]
  "Counts (map)" <- w7
  n8 = call <vilib>:"Histogram.vi"("intervals"=255, "X"=w14) -> ("Histogram Graph"=→"Histogram Graph":T1)  [unwired: 5 in, 4 out]
  n9 = Split 1D Array(array=w44, index=5) -> (first subarray=w42:u8[], second subarray=w38:u8[])
  n10 = for {
    tunnel: w7 -> [w50] mode=indexing
    tunnel: [w49] -> w6 mode=indexing
    tunnel: [w48] -> w5 mode=indexing
    n11 = Unbundle(w50) -> ("key"=w49:u32, "value"=w48:u32)
  }
  n12 = Collection Size(1:w7) -> (0:w8:i32)
  n13 = Byte Array To String(unsigned byte array=w42) -> (string=w39:string)
  n14 = Split 1D Array(array=w38, index=12) -> (first subarray=w35:u8[], second subarray=w31:u8[])
  n15 = Reverse String(1:w39) -> (0:w19:string)
  n16 = Decrement(x=w8) -> (x-1=w9:i32)
  n17 = Byte Array To String(unsigned byte array=w35) -> (string=w36:string)
  n18 = Split 1D Array(array=w31, index=8) -> (first subarray=w32:u8[])  [unwired: 1 out]
  n19 = for {
    N: w9 -> [w58]
    shift-right: [w52] -> w4
    shift-left: w5 -> [w53]
    shift-right: [w51] -> w2
    shift-left: w6 -> [w54]
    i -> [w57]
    n20 = Subtract(x=w58, y=w57) -> (x-y=w56:i32)
    n21 = Decrement(x=w56) -> (x-1=w55:i32)
    n22 = for {
      N: w55 -> [_]
      shift-right: [w60] -> w52
      shift-left: w53 -> [w61]
      shift-right: [w59] -> w51
      shift-left: w54 -> [w64]
      i -> [w63]
      n23 = Increment(x=w63) -> (x+1=w62:i32)
      n24 = in-place {
        n25 = in-place-array #1(w61, w63) -> (w72:u32)
        n26 = in-place-array #2(w61, w62) -> (w71:u32)
        n27 = in-place-array #3(w64, w63) -> (w68:u32)
        n28 = in-place-array #4(w64, w62) -> (w67:u32)
        n29 = Greater?(x=w72, y=w71) -> (0:w69:bool)
        n30 = Select(t=w68, s=w69, f=w67) -> (s? t:f=w65:u32)
        n31 = Select(t=w67, s=w69, f=w68) -> (s? t:f=w66:u32)
        n32 = Select(t=w71, s=w69, f=w72) -> (s? t:f=w73:u32)
        n33 = Select(t=w72, s=w69, f=w71) -> (s? t:f=w70:u32)
        n34 = in-place-array #1(w73) -> (w60:u32[])  [unwired: 1 out]
        n35 = in-place-array #2(w70) -> ()  [unwired: 2 out]
        n36 = in-place-array #3(w66) -> (w59:u32[])  [unwired: 1 out]
        n37 = in-place-array #4(w65) -> ()  [unwired: 2 out]
      }
    }
  }
  n38 = Scan Value(string=w19, format string="%b", default (0 dbl)=u32 0) -> (value=→"rsvd+partity":u32)  [unwired: 1 out]
  n39 = Reverse String(1:w36) -> (0:w23:string)
  n40 = Byte Array To String(unsigned byte array=w32) -> (string=w33:string)
  n41 = Reverse String(1:w33) -> (0:w30:string)
  n42 = Scan Value(string=w23, format string="%b", default (0 dbl)=u32 0) -> (value=→"pha":u32)  [unwired: 1 out]
  n43 = Scan Value(string=w30, format string="%b", default (0 dbl)=u32 0) -> (value=→"channel":u32)  [unwired: 1 out]
  n44 = Reverse 1D Array(array=w4) -> (reversed array=→"Value sort":u32[])
  n45 = Reverse 1D Array(array=w2) -> (reversed array=→"key sort":u32[])
